vi "运维调试_五参数.vi"() -> ()   [LabVIEW 2016, in "斯坦道原位多参数.lvlib"]
uses:
  <vilib>/Utility/miscctls.llb/LVPointTypeDef.ctl
  <vilib>/Utility/config.llb/NI_LVConfig.lvlib
panel:
  in  "获取传感器参数并保存触发":bool
  in  "传感器参数自动获取":bool=TRUE
  in  "标样测试组数":dbl=1.0 caption="标样测试组数:"
  in  "水样测试组数":dbl=1.0 caption="水样测试组数:"
  in  "转刷清洗时间":dbl=30.0 caption="转刷清洗时间:"
  in  "上电初始化时间":dbl=5.0 caption="上电初始化时间:"
  in  "水样稳定时间":dbl=5.0 caption="水样稳定时间:"
  out "串口号":string
  in  "水深写入":bool
  in  "水深读取":bool
  in  "水深校准":dbl caption="水深校准:"
  out "模块版本号":string
  in  "写入":bool
  in  "读取":bool
  in  "B":dbl caption="校准值B:"
  in  "K":dbl caption="校准值K:"
  in  "标样核查":bool
  in  "串口设置":bool
  in  "质控参数设置":bool
  in  "打开串口":bool
  in  "释放串口":bool
  out "多参数横条运行状态":T1(xcontrol)
  in  "数据区":i32(listbox)
  in  "停止测量(单探)":bool
  in  "启动测量(单探)":bool
  in  "控制命令区探头选择":u16(ring)=9 items=["氨氮"=3, "水温"=9, "pH值"=10, "溶解氧"=11, "电导率"=12, "浊度"=13, "叶绿素a"=14, "藻密度"=15, "蓝绿藻"=16, "氧化还原电位"=17, "溶解氧%"=18, "盐度"=19]
  in  "同步时间":bool
  in  "初始化(清洗)":bool
  in  "停止测量(全部)":bool
  in  "启动测量(全部)":bool
  in  "关键参数区读取":bool
  in  "关键参数区":i32(listbox)
  in  "传感器参数读取":bool
  in  "传感器区":i32(listbox)
  in  "返回":bool
  in  "设置":bool
  out "运行状态":string
  in  "停止":bool
  in  "水样测试":bool
  out "集成报警信息":string
  # "min"
  # "组"
  # "组"
  # "s"
  # "s"
  # "控制命令区"
  # "探头校准"
  # "水深校准"
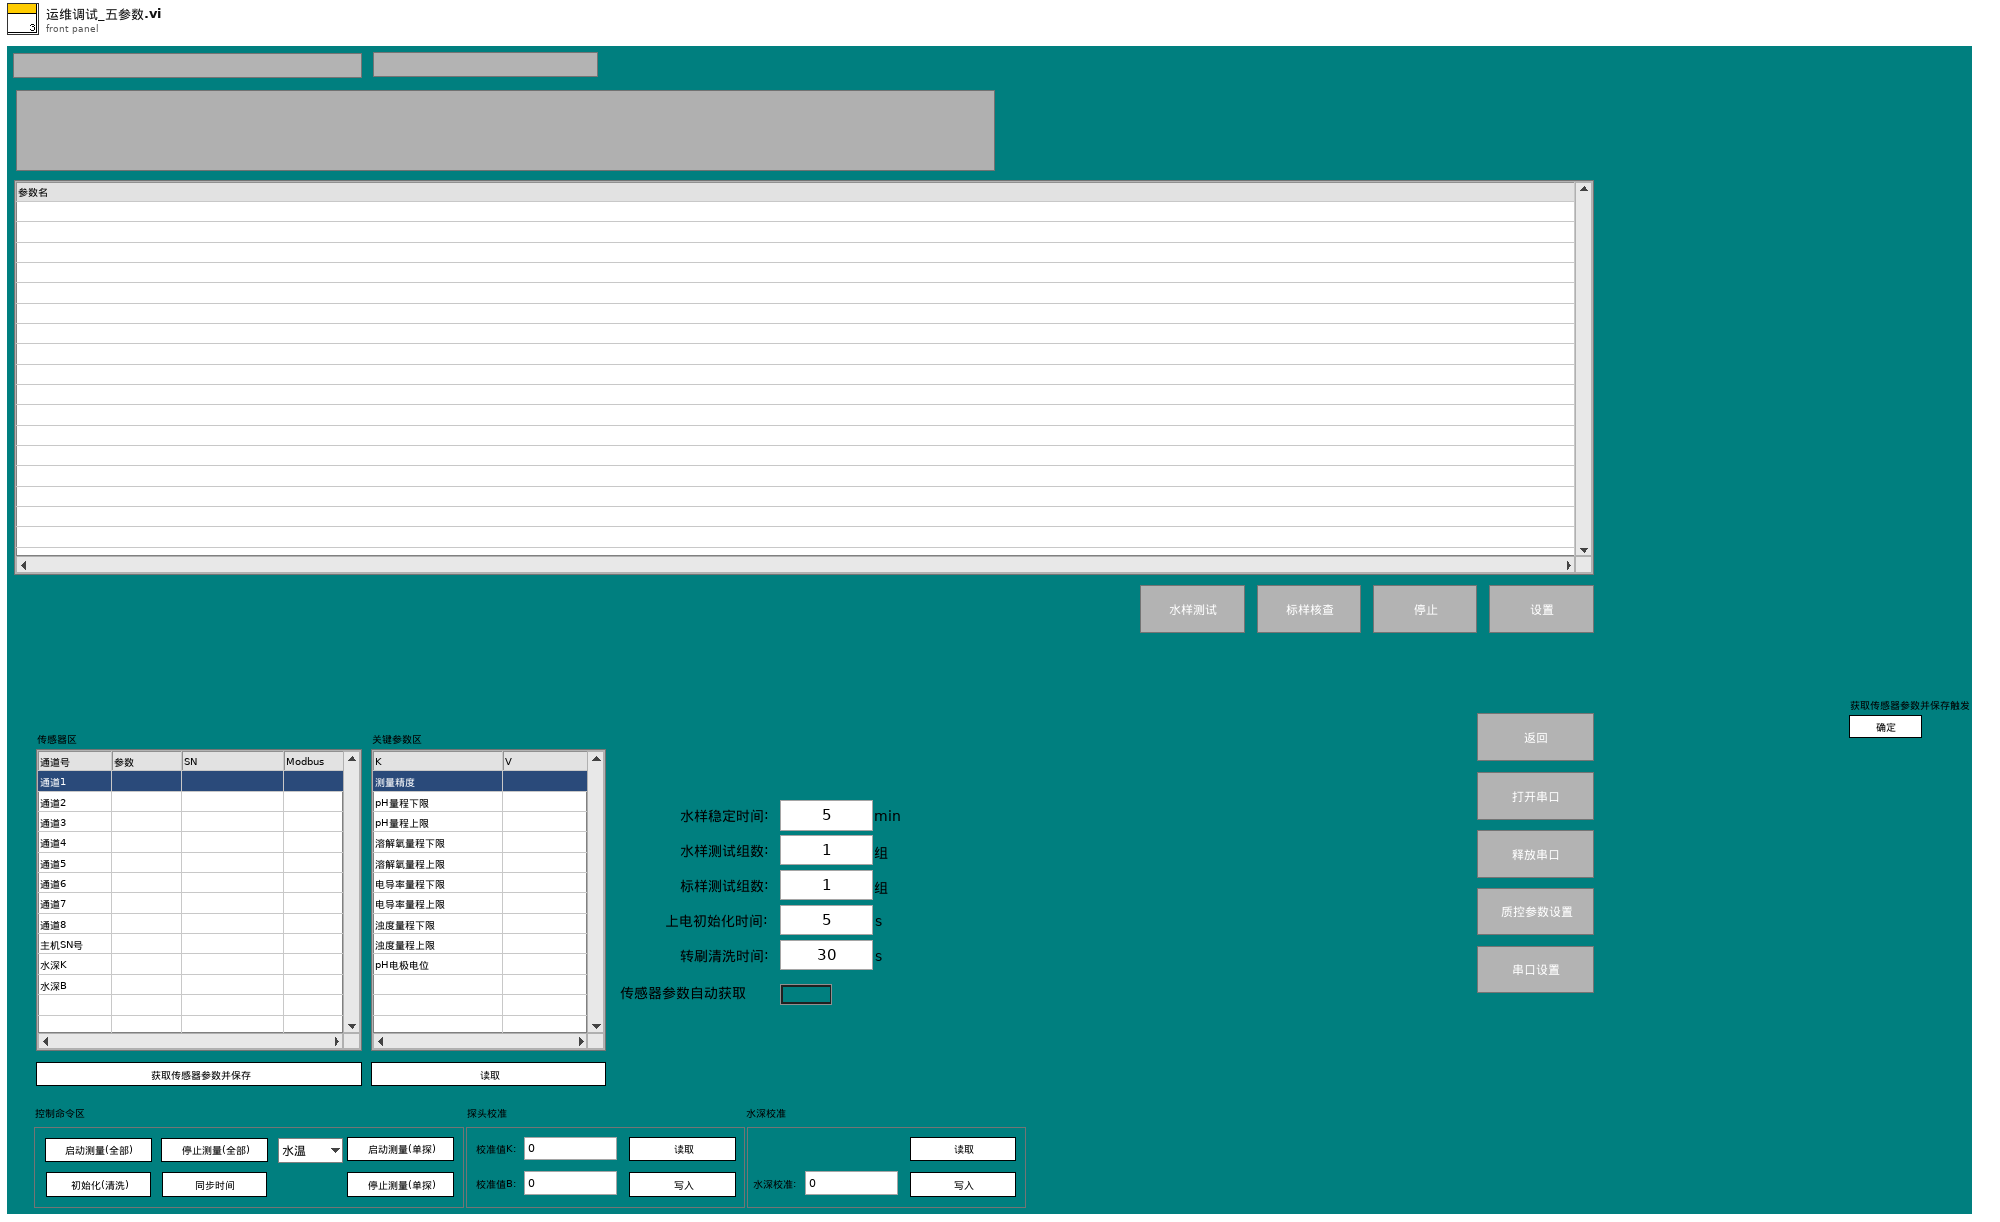
[diagram p1: front panel]
types:
  T1 = cluster{"系统时间":timestamp, "工作状态":u16, "测量模式":u16, "告警代码":enum16{"无告警", "缺试剂告警", "缺水样告警", "缺蒸馏水告警", "缺标液告警", "仪表漏液告警", "标定异常告警", "超量程告警", "加热异常", "低试剂预警", "超上限告警", "超下限告警", "仪表内部其他异常", "滴定异常告警", "电极异常告警", "量程切换告警", "参数设置告警", "PH电极电位异常", "电导率电极异常", "浊度光度异常", "溶解氧电极异常", "溶解氧光强异常", "温度异常告警", "PH异常告警", "溶解氧异常告警", "电导率异常告警", "浊度异常告警", "叶绿素异常告警", "藻密度异常告警", "蓝绿藻异常告警", "ORP异常告警", "氨氮异常告警", "清洁刷异常告警", "SD卡异常告警", "蓝牙异常告警", "Wifi异常告警", "流程异常告警"}, "故障代码":enum16{"无故障", "电机故障", "温度故障", "通讯故障", "滴定故障"}, "日志代码":u16, "软件版本":string}
  T2 = typedef "斯坦道原位多参数.lvlib/水样测试启动自定义输入参数.ctl" = cluster{"测量模式":string, "数据类型":string}
  T3 = typedef "LVPointTypeDef.ctl" = cluster{"Horizontal":i16, "Vertical":i16}
  T4 = typedef "报警信息字段定义.ctl" = cluster{"时间":timestamp, "参数":string, "报警信息":string, "备注":string}
  T5 = enum16{"无告警", "缺试剂告警", "缺水样告警", "缺蒸馏水告警", "缺标液告警", "仪表漏液告警", "标定异常告警", "超量程告警", "加热异常", "低试剂预警", "超上限告警", "超下限告警", "仪表内部其他异常", "滴定异常告警", "电极异常告警", "量程切换告警", "参数设置告警", "PH电极电位异常", "电导率电极异常", "浊度光度异常", "溶解氧电极异常", "溶解氧光强异常", "温度异常告警", "PH异常告警", "溶解氧异常告警", "电导率异常告警", "浊度异常告警", "叶绿素异常告警", "藻密度异常告警", "蓝绿藻异常告警", "ORP异常告警", "氨氮异常告警", "清洁刷异常告警", "SD卡异常告警", "蓝牙异常告警", "Wifi异常告警", "流程异常告警"}
  T6 = cluster{"水温":dbl, "pH":dbl, "DO":dbl, "Cond":dbl, "Turb":dbl, "叶绿素":dbl, "藻密度":dbl, "蓝绿藻":dbl, "ORP":dbl, "NH3N":dbl}
  T7 = cluster{"因子编码":string, "单位":string, "标样参考值":sgl, "水样数据时间":timestamp, "水样实测值":sgl, "水样数据标识":string, "K":sgl, "B":sgl, "T":sgl, "H":sgl, "水深":sgl, "探头温度":sgl}
  T8 = cluster{"Major":u16, "Minor":u16, "Fix":u16, "Build":u16}
  T9 = typedef "NI_LVConfig.lvlib/Config Data RefNum.ctl" = refnum<k1>
  T10 = enum8{"Enabled", "Disabled", "Disabled and Grayed Out"}
  T11 = typedef "斯坦道原位多参数.lvlib/标样核查启动自定义输入参数.ctl" = cluster{"测量模式":string, "数据类型":string, "输出参数":cluster{"水温":bool, "pH":bool, "DO":bool, "浊度":bool, "电导率":bool}}
  T12 = cluster{"水温标准液标准浓度":dbl, "酸碱度标准液标准浓度":dbl, "溶解氧标准液标准浓度":dbl, "电导率标准液标准浓度":dbl, "浊度标准液标准浓度":dbl}
  T13 = cluster{"确定":bool, "水温标准液标准浓度":dbl, "酸碱度标准液标准浓度":dbl, "溶解氧标准液标准浓度":dbl, "电导率标准液标准浓度":dbl, "浊度标准液标准浓度":dbl}
  T14 = cluster{"运行模式":enum16{"维护模式", "常规模式", "应急模式", "质控模式"}, "24H周期设置":bool[]}
  T15 = cluster{"水温":bool, "pH":bool, "DO":bool, "浊度":bool, "电导率":bool}
  T16 = enum32{"Bad", "Idle", "Run top level", "Running"}
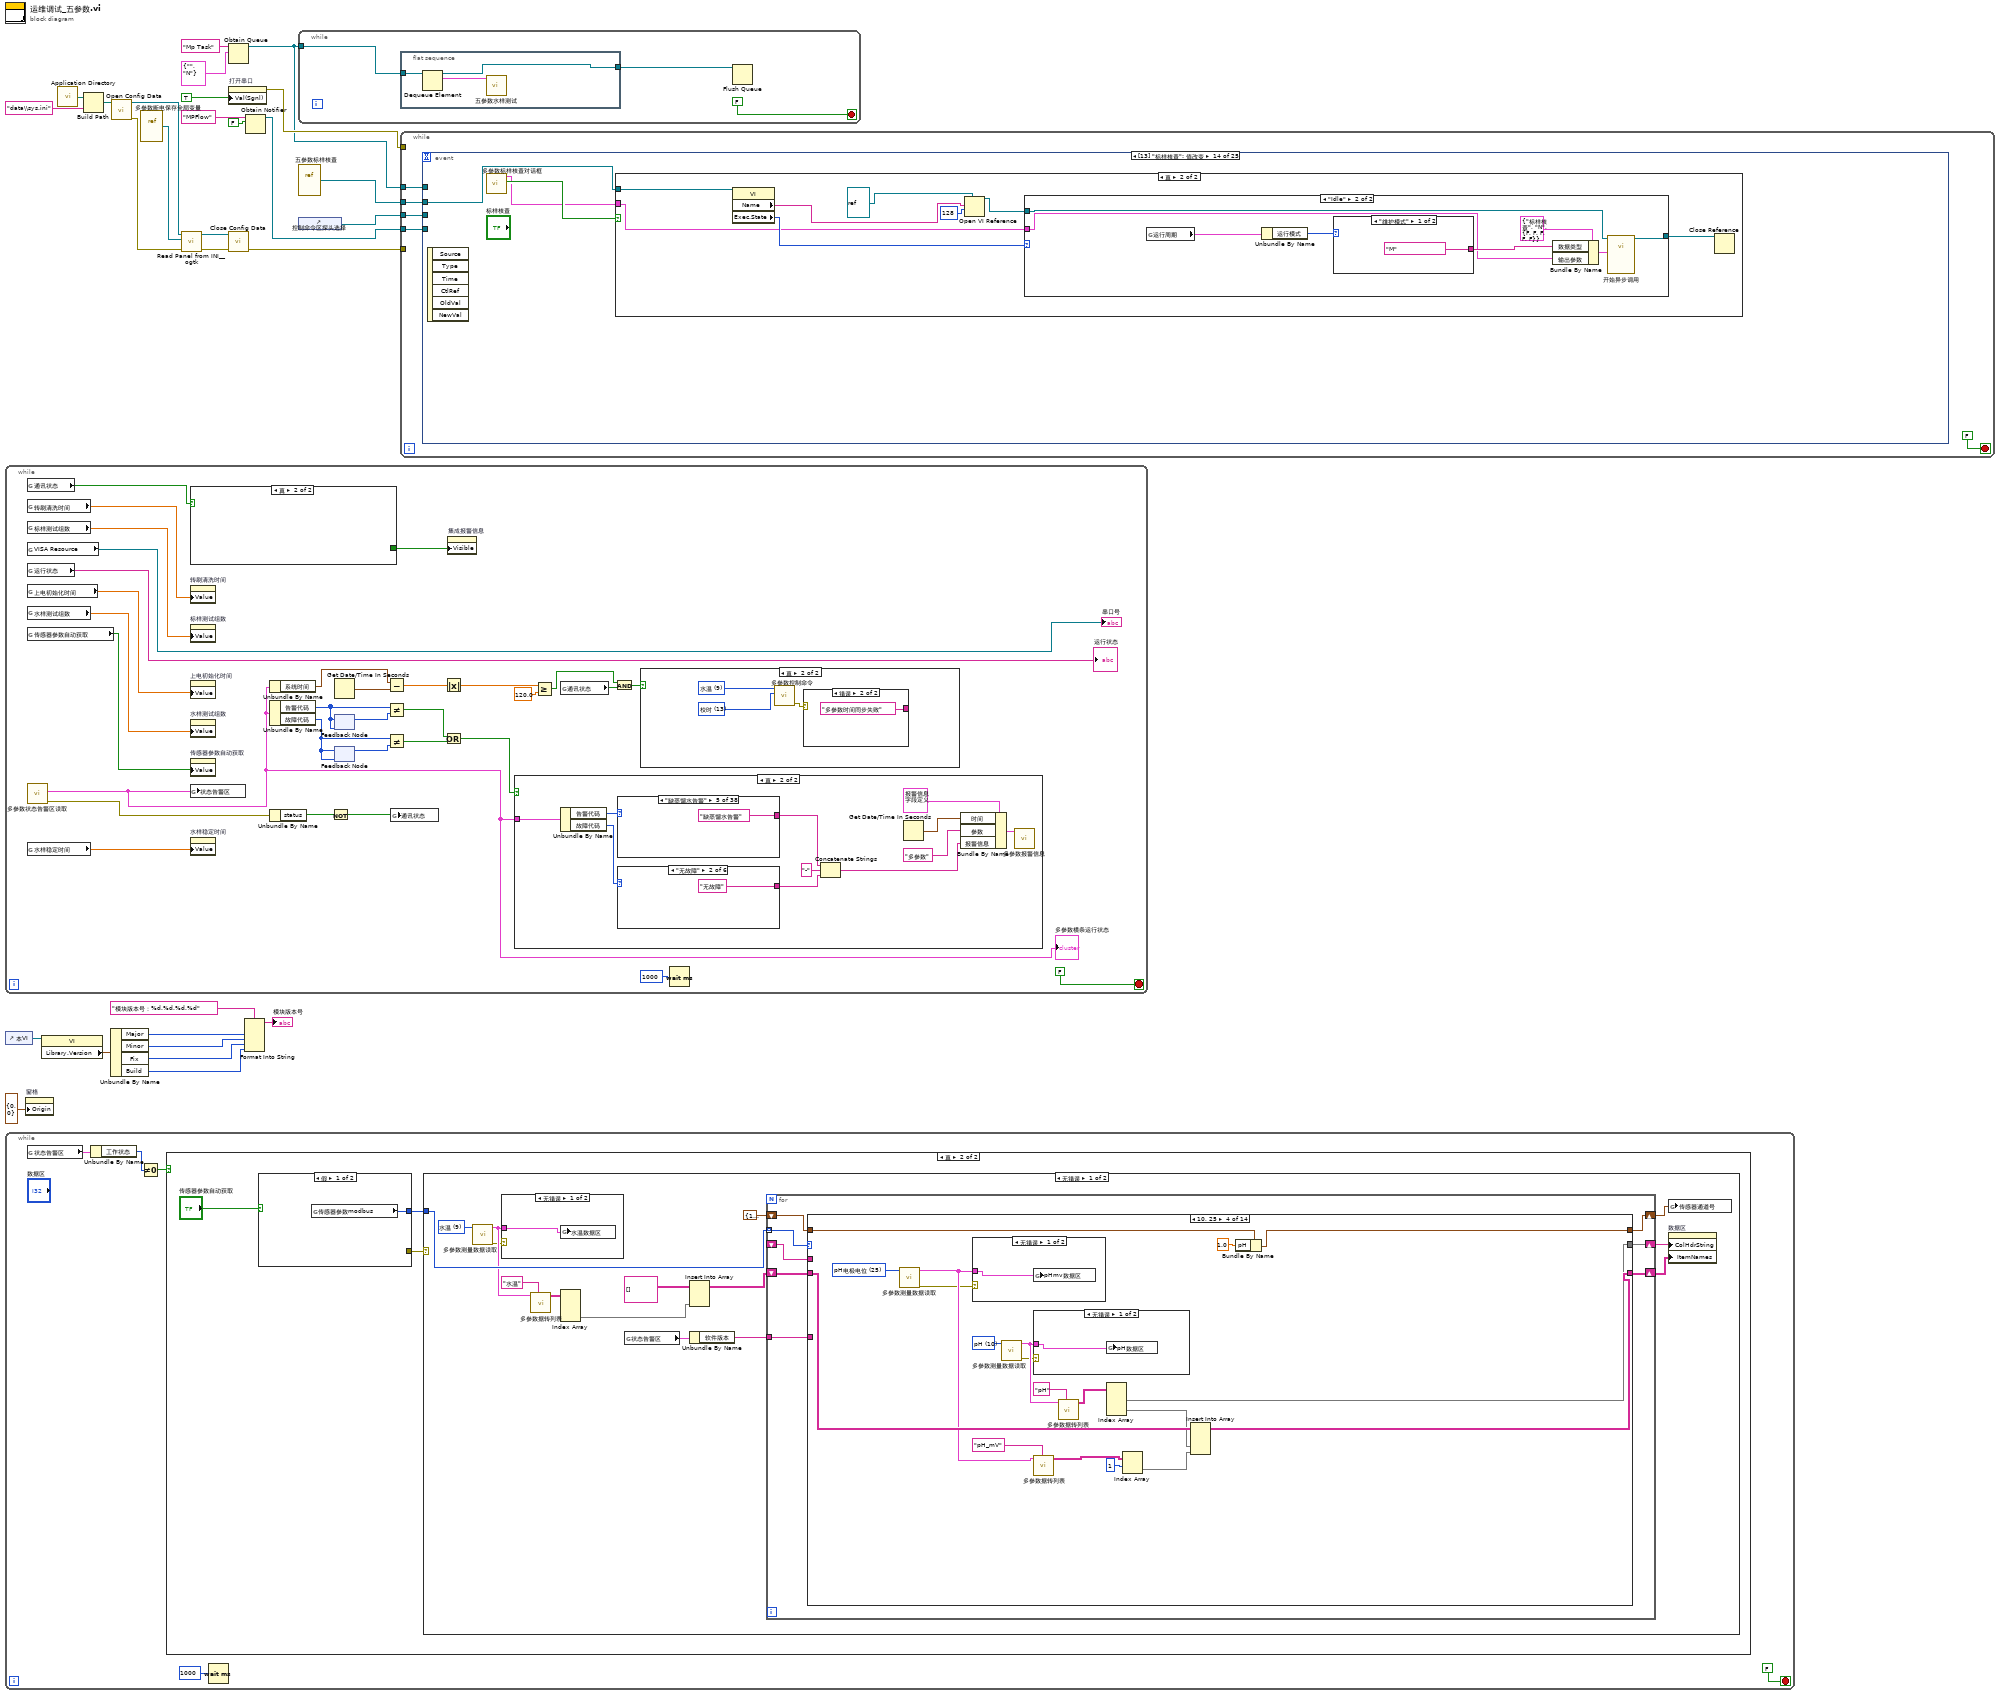
[diagram p0: block diagram]
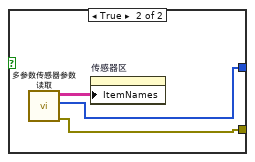
[diagram p3: hidden frame]
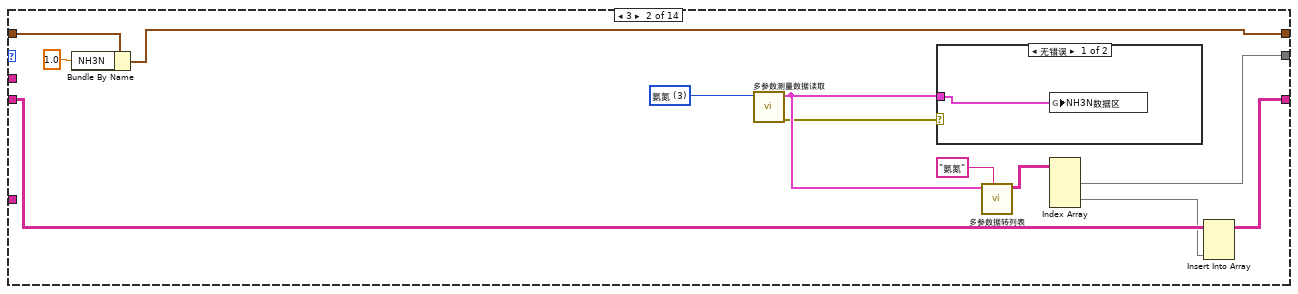
[diagram p6: hidden frame]
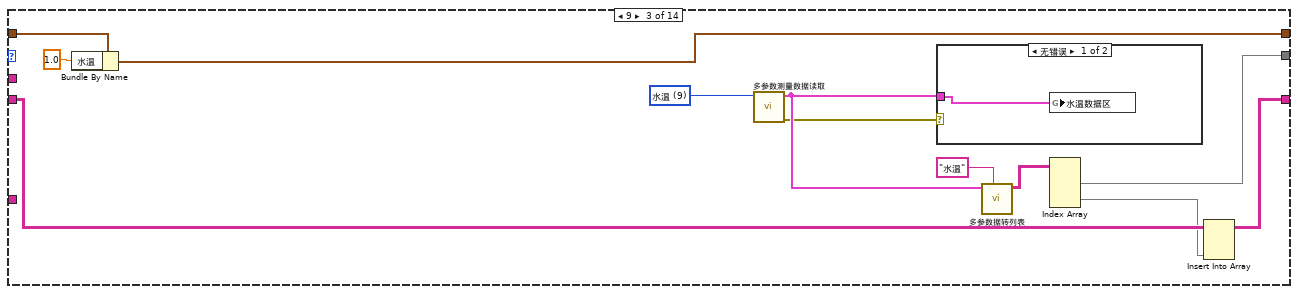
[diagram p8: hidden frame]
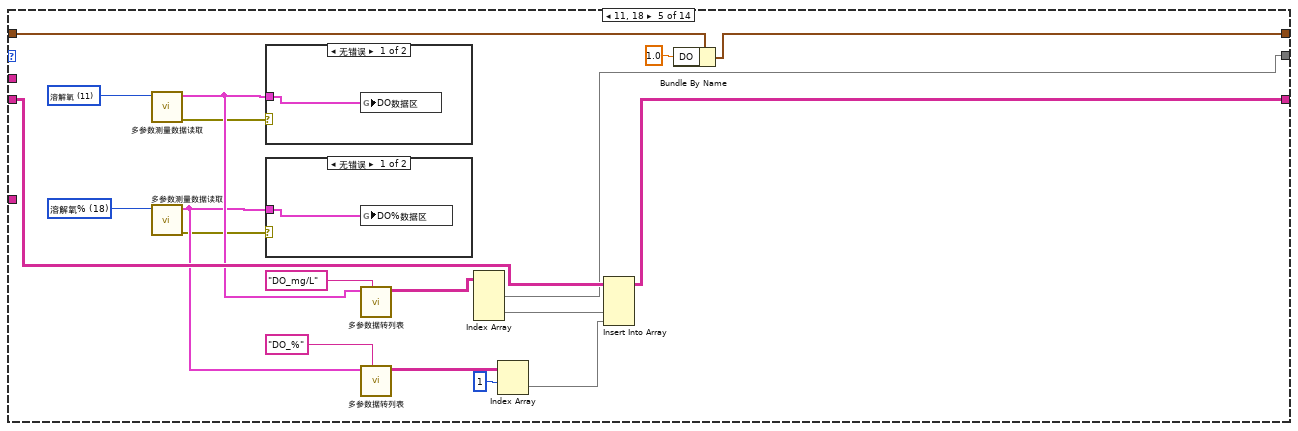
[diagram p12: hidden frame]
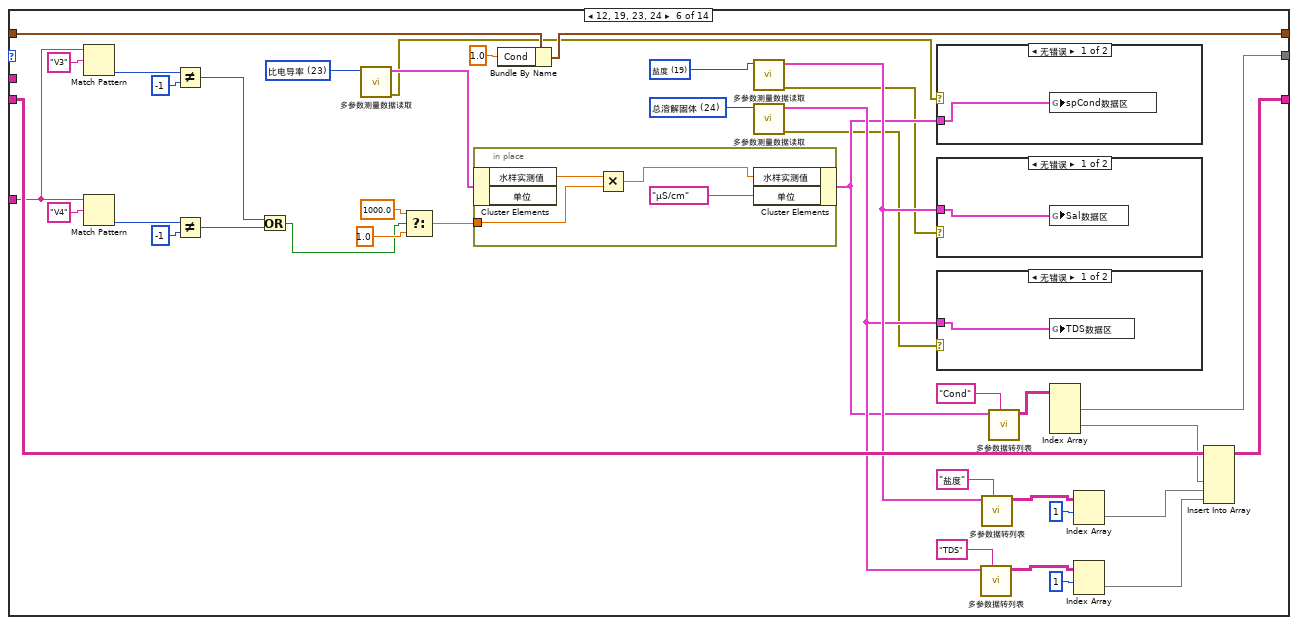
[diagram p15: hidden frame]
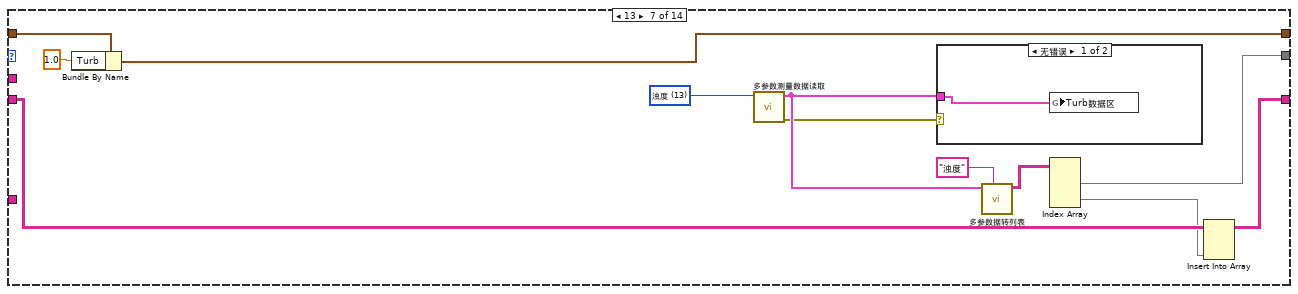
[diagram p19: hidden frame]
diagram:
  n1 = while {
    stop <- FALSE stop-if-true
    n2 = global read "多参数全局变量.vi" "通讯状态"() -> (w57:bool)
    n3 = global read "多参数断电保存全局变量.vi" "转刷清洗时间"() -> (w31:dbl)
    n4 = global read "多参数断电保存全局变量.vi" "标样测试组数"() -> (w30:dbl)
    n5 = global read "多参数断电保存全局变量.vi" "VISA Resource"() -> (→"串口号":refnum<visa-resource-name>)
    n6 = global read "多参数全局变量.vi" "运行状态"() -> (→"运行状态":string)
    n7 = global read "多参数断电保存全局变量.vi" "上电初始化时间"() -> (w32:dbl)
    n8 = global read "多参数断电保存全局变量.vi" "水样测试组数"() -> (w33:dbl)
    n9 = global read "多参数断电保存全局变量.vi" "传感器参数自动获取"() -> (w29:bool)
    n10 = call "多参数状态告警区读取.vi"() -> ("error out"=w47:errorcluster, "状态告警块"=w44:T1)  [unwired: 9 in, 1 out]
    "多参数横条运行状态" <- w44
    n11 = global read "多参数断电保存全局变量.vi" "水样稳定时间"() -> (w34:dbl)
    n12 = case shown="真" w57 {
      tunnel: [TRUE ("可见") _] -> w56
      frame False {
        "集成报警信息" <- "通讯异常" ("集成报警信息")
      }
      frame True {
      }
    }
    n13 = property on="转刷清洗时间" class="DigNum (严格)"("Value"=w31) -> ()  [unwired: 2 in, 2 out]
    n14 = property on="标样测试组数" class="DigNum (严格)"("Value"=w30) -> ()  [unwired: 2 in, 2 out]
    n15 = property on="上电初始化时间" class="DigNum (严格)"("Value"=w32) -> ()  [unwired: 2 in, 2 out]
    n16 = property on="水样测试组数" class="DigNum (严格)"("Value"=w33) -> ()  [unwired: 2 in, 2 out]
    n17 = property on="传感器参数自动获取" class="Bool (严格)"("Value"=w29) -> ()  [unwired: 2 in, 2 out]
    n18 = global write "多参数全局变量.vi" "状态告警区"(w44) -> ()
    n19 = property on="水样稳定时间" class="DigNum (严格)"("Value"=w34) -> ()  [unwired: 2 in, 2 out]
    n20 = Unbundle By Name(w44) -> ("系统时间"=w43:timestamp)
    n21 = Unbundle By Name(w44) -> ("告警代码"=w53:T5, "故障代码"=w51:enum16{"无故障", "电机故障", "温度故障", "通讯故障", "滴定故障"})
    n22 = Unbundle By Name(w47) -> ("status"=w46:bool)
    n23 = Not(x=w46) -> (.not. x?=w45:bool)
    n24 = Get Date/Time In Seconds() -> (seconds since 1Jan1904=w42:timestamp)
    n25 = feedback #1(w53) -> (w54:T5)
    n26 = feedback-in #1(w53) -> ()
    n27 = feedback #2(w51) -> (w52:enum16{"无故障", "电机故障", "温度故障", "通讯故障", "滴定故障"})
    n28 = feedback-in #2(w51) -> ()
    n29 = Subtract(x=w43, y=w42) -> (x-y=w41:dbl)
    n30 = Not Equal?(x=w53, y=w54) -> (x != y?=w49:bool)
    n31 = Not Equal?(x=w51, y=w52) -> (x != y?=w50:bool)
    n32 = global write "多参数全局变量.vi" "通讯状态"(w45) -> ()
    n33 = Absolute Value(x=w41) -> (abs(x)=w40:dbl)
    n34 = Or(x=w49, y=w50) -> (x .or. y?=w48:bool)
    n35 = property on="集成报警信息" class="Str"("Visible"=w56) -> ()  [unwired: 2 in, 2 out]
    n36 = case shown="真" w48 {
      tunnel: w44 -> [_ w75]
      frame False {
      }
      frame True {
        n37 = Unbundle By Name(w75) -> ("告警代码"=w74:T5, "故障代码"=w73:enum16{"无故障", "电机故障", "温度故障", "通讯故障", "滴定故障"})
        n38 = case shown="\"缺蒸馏水告警\"" w74 {
          selector: w74 -> [w86 _ _ _ _ _ _ _ _ _ _ _ _ _ _ _ _ _ _ _ _ _ _ _ _ _ _ _ _ _ _ _ _ _ _ _ _ _]
          tunnel: [w85 "无告警" "缺试剂告警" "缺水样告警" "缺蒸馏水告警" "缺标液告警" "仪表漏液告警" "标定异常告警" "超量程告警" "加热异常" "低试剂预警" "超上限告警" "超下限告警" "仪表内部其他异常" "滴定异常告警" "电极异常告警" "量程切换告警" "参数设置告警" "PH电极电位异常" "电导率电极异常" "浊度光度异常" "溶解氧电极异常" "溶解氧光强异常" "温度异常告警" "PH异常告警" "溶解氧异常告警" "电导率异常告警" "浊度异常告警" "叶绿素异常告警" "藻密度异常告警" "蓝绿藻异常告警" "ORP异常告警" "氨氮异常告警" "清洁刷异常告警" "SD卡异常告警" "蓝牙异常告警" "WiFi异常告警" "流程异常告警"] -> w72
          frame Default {
            n39 = Format Into String(format string="%d" ("格式字符串"), initial string="未知" ("工作状态"), w86) -> (resulting string=w85:string)  [unwired: 1 in, 1 out]
          }
          frame "无告警" {
          }
          frame "缺试剂告警" {
          }
          frame "缺水样告警" {
          }
          frame "缺蒸馏水告警" {
          }
          frame "缺标液告警" {
          }
          frame "仪表漏液告警" {
          }
          frame "标定异常告警" {
          }
          frame "超量程告警" {
          }
          frame "加热异常" {
          }
          frame "低试剂预警" {
          }
          frame "超上限告警" {
          }
          frame "超下限告警" {
          }
          frame "仪表内部其他异常" {
          }
          frame "滴定异常告警" {
          }
          frame "电极异常告警" {
          }
          frame "量程切换告警" {
          }
          frame "参数设置告警" {
          }
          frame "PH电极电位异常" {
          }
          frame "电导率电极异常" {
          }
          frame "浊度光度异常" {
          }
          frame "溶解氧电极异常" {
          }
          frame "溶解氧光强异常" {
          }
          frame "温度异常告警" {
          }
          frame "PH异常告警" {
          }
          frame "溶解氧异常告警" {
          }
          frame "电导率异常告警" {
          }
          frame "浊度异常告警" {
          }
          frame "叶绿素异常告警" {
          }
          frame "藻密度异常告警" {
          }
          frame "蓝绿藻异常告警" {
          }
          frame "ORP异常告警" {
          }
          frame "氨氮异常告警" {
          }
          frame "清洁刷异常告警" {
          }
          frame "SD卡异常告警" {
          }
          frame "蓝牙异常告警" {
          }
          frame "Wifi异常告警" {
          }
          frame "流程异常告警" {
          }
        }
        n40 = case shown="\"无故障\"" w73 {
          selector: w73 -> [w77 _ _ _ _ _]
          tunnel: [w76 "无故障" "电机故障" "温度故障" "通讯故障" "滴定故障"] -> w71
          frame Default {
            n41 = Format Into String(format string="%d" ("格式字符串"), initial string="未知" ("工作状态"), w77) -> (resulting string=w76:string)  [unwired: 1 in, 1 out]
          }
          frame "无故障" {
          }
          frame "电机故障" {
          }
          frame "温度故障" {
          }
          frame "通讯故障" {
          }
          frame "滴定故障" {
          }
        }
        n42 = Concatenate Strings(w72, "-" ("字符串"), w71) -> (w69:string)
        n43 = Get Date/Time In Seconds() -> (seconds since 1Jan1904=w68:timestamp)
        n44 = Bundle By Name(cluster=T4 {"时间"=timestamp(0 s since 1904-01-01), "参数"="", "报警信息"="", "备注"=""} ("data"), "时间"=w68, "参数"="多参数" ("设备"), "报警信息"=w69) -> (w65:T4)
        n45 = call "多参数报警信息.vi"("data"=w65) -> ()  [unwired: 10 in, 1 out]
      }
    }
    n46 = Greater Or Equal?(x=w40, y=120.0) -> (x >= y?=w39:bool)
    n47 = global read "多参数全局变量.vi" "通讯状态"() -> (w36:bool)
    n48 = And(x=w39, y=w36) -> (x .and. y?=w37:bool)
    n49 = case shown="真" w37 {
      frame False {
      }
      frame True {
        w60 = u16 13 items=["启动测量（全部）"=1, "初始化（清洗）"=10, "停止测量（全部）"=11, "校时"=13, "启动测量（单个传感器）"=19, "停止测量（单个传感器）"=20] ("控制命令")
        w61 = u16 9 items=["氨氮"=3, "水温"=9, "pH值"=10, "溶解氧"=11, "电导率"=12, "浊度"=13, "叶绿素a"=14, "藻密度"=15, "蓝绿藻"=16, "氧化还原电位"=17, "溶解氧%"=18, "盐度"=19] ("站号")
        n50 = call "多参数控制命令.vi"("控制命令"=w60, "站号"=w61) -> ("error out"=w62:errorcluster)  [unwired: 9 in]
        n51 = case shown="错误" w62 {
          tunnel: ["多参数时间同步成功" ("消息") "多参数时间同步失败" ("消息")] -> _
          frame No Error {
          }
          frame Error {
          }
        }
      }
    }
    n52 = Wait (ms)(milliseconds to wait=u32 1000 ("等待时间（毫秒）")) -> ()  [unwired: 1 out]
  }
  n53 = control-ref of="本VI"() -> (w8:refnum<vi>)
  n54 = while {
    stop <- FALSE stop-if-true
    n55 = global read "多参数全局变量.vi" "状态告警区"() -> (w130:T1)
    n56 = Unbundle By Name(w130) -> ("工作状态"=w129:u16)
    n57 = Not Equal To 0?(x=w129) -> (x != 0?=w128:bool)
    n58 = case shown="真" w128 {
      frame False {
      }
      frame True {
        n59 = case shown="假" "传感器参数自动获取" {
          tunnel: [_ w139] -> w135
          tunnel: [w136 w138] -> w134
          frame False {
            n60 = global read "多参数断电保存全局变量.vi" "传感器参数modbus"() -> (w136:u16[])
          }
          frame True {
            n61 = call "多参数传感器参数读取.vi"() -> ("error out"=w139:errorcluster, "modbus"=w138:u16[], "添加的数组"=w137:string[][])  [unwired: 9 in]
            n62 = property on="传感器区" class="MCListbox (严格)"("ItemNames"=w137) -> ()  [unwired: 2 in, 2 out]
          }
        }
        n63 = case shown="无错误" w135 {
          tunnel: w134 -> [w154 _]
          frame No Error {
            w151 = u16 9 items=["氨氮"=3, "水温"=9, "pH"=10, "溶解氧"=11, "电导率"=12, "浊度"=13, "叶绿素a"=14, "藻密度"=15, "蓝绿藻"=16, "氧化还原电位"=17, "溶解氧%"=18, "盐度"=19, "水中油"=20, "高锰酸盐指数"=21, "化学需氧量"=22, "比电导率"=23, "总溶解固体"=24, "pH电极电位"=25] ("下拉列表")
            n64 = call "多参数测量数据读取.vi"("探头选择"=w151) -> ("error out"=w140:errorcluster, "测量数据块"=w146:T7)  [unwired: 8 in, 1 out]
            n65 = case shown="无错误" w140 {
              tunnel: w146 -> [w155 _]
              frame No Error {
                n66 = global write "多参数全局变量.vi" "水温数据区"(w155) -> ()
              }
              frame Error {
              }
            }
            n67 = call "多参数据转列表.vi"("参数名"="水温", "测量数据块"=w146) -> ("添加的数组"=w144:string[][])  [unwired: 9 in]
            n68 = Index Array(array=w144) -> (element #2=w143:string[])  [unwired: 4 in, 1 out]
            n69 = global read "多参数全局变量.vi" "状态告警区"() -> (w142:T1)
            n70 = Insert Into Array(array=string[][] [] ("子数组"), new element=w143) -> (w149:string[][])  [unwired: 2 in]
            n71 = Unbundle By Name(w142) -> ("软件版本"=w141:string)
            n72 = for {
              tunnel: w154 -> [w163] mode=indexing
              shift-right: [w161] -> w152
              shift-left: w149 -> [w162]
              shift-right: [w160] -> w153
              shift-left: _ -> [w159]
              shift-right: [w158] -> w147
              shift-left: T6 {"水温"=1.0, "pH"=0.0, "DO"=0.0, "Cond"=0.0, "Turb"=0.0, "叶绿素"=0.0, "藻密度"=0.0, "蓝绿藻"=0.0, "ORP"=0.0, "NH3N"=0.0} ("传感器通道号") -> [w157]
              tunnel: w141 -> [w156]
              n73 = case shown="10, 25" w163 {
                tunnel: w162 -> [w166 w177 w190 w210 w231 w273 w292 w305 w318 w331 w344 w354 w363 w372]
                tunnel: [w166 w176 w189 w209 w230 w272 w291 w304 w317 w330 w343 w353 w362 w371] -> w161
                tunnel: [w165 w169 w182 w202 w223 w264 w285 w297 w312 w324 w337 w348 w357 w366] -> w160
                tunnel: w159 -> [w165 _ _ _ _ _ _ _ _ _ _ _ _ _]
                tunnel: [w164 w173 w186 w205 w227 w267 w288 w301 w314 w327 w340 w352 w361 w370] -> w158
                tunnel: w157 -> [w164 w175 w188 w207 w229 w268 w289 w302 w315 w328 w341 w352 w361 w370]
                tunnel: w156 -> [_ _ _ _ _ w243 _ _ _ _ _ _ _ _]
                frame 0, Default {
                }
                frame 3 {
                  w178 = u16 3 items=["氨氮"=3, "水温"=9, "pH"=10, "溶解氧"=11, "电导率"=12, "浊度"=13, "叶绿素a"=14, "藻密度"=15, "蓝绿藻"=16, "氧化还原电位"=17, "溶解氧%"=18, "盐度"=19, "水中油"=20, "高锰酸盐指数"=21, "化学需氧量"=22, "比电导率"=23, "总溶解固体"=24, "pH电极电位"=25] ("下拉列表")
                  n74 = Bundle By Name(cluster=w175, "NH3N"=1.0) -> (w173:T6)
                  n75 = call "多参数测量数据读取.vi"("探头选择"=w178) -> ("error out"=w167:errorcluster, "测量数据块"=w172:T7)  [unwired: 8 in, 1 out]
                  n76 = case shown="无错误" w167 {
                    tunnel: w172 -> [w179 _]
                    frame No Error {
                      n77 = global write "多参数全局变量.vi" "NH3N数据区"(w179) -> ()
                    }
                    frame Error {
                    }
                  }
                  n78 = call "多参数据转列表.vi"("参数名"="氨氮", "测量数据块"=w172) -> ("添加的数组"=w171:string[][])  [unwired: 9 in]
                  n79 = Index Array(array=w171) -> (element #1=w169:string[], element #2=w168:string[])  [unwired: 4 in]
                  n80 = Insert Into Array(array=w177, new element=w168) -> (w176:string[][])  [unwired: 2 in]
                }
                frame 9 {
                  w191 = u16 9 items=["氨氮"=3, "水温"=9, "pH"=10, "溶解氧"=11, "电导率"=12, "浊度"=13, "叶绿素a"=14, "藻密度"=15, "蓝绿藻"=16, "氧化还原电位"=17, "溶解氧%"=18, "盐度"=19, "水中油"=20, "高锰酸盐指数"=21, "化学需氧量"=22, "比电导率"=23, "总溶解固体"=24, "pH电极电位"=25] ("下拉列表")
                  n81 = Bundle By Name(cluster=w188, "水温"=1.0) -> (w186:T6)
                  n82 = call "多参数测量数据读取.vi"("探头选择"=w191) -> ("error out"=w180:errorcluster, "测量数据块"=w185:T7)  [unwired: 8 in, 1 out]
                  n83 = case shown="无错误" w180 {
                    tunnel: w185 -> [w192 _]
                    frame No Error {
                      n84 = global write "多参数全局变量.vi" "水温数据区"(w192) -> ()
                    }
                    frame Error {
                    }
                  }
                  n85 = call "多参数据转列表.vi"("参数名"="水温", "测量数据块"=w185) -> ("添加的数组"=w184:string[][])  [unwired: 9 in]
                  n86 = Index Array(array=w184) -> (element #1=w182:string[], element #2=w181:string[])  [unwired: 4 in]
                  n87 = Insert Into Array(array=w190, new element=w181) -> (w189:string[][])  [unwired: 2 in]
                }
                frame 10, 25 {
                  w208 = u16 25 items=["氨氮"=3, "水温"=9, "pH"=10, "溶解氧"=11, "电导率"=12, "浊度"=13, "叶绿素a"=14, "藻密度"=15, "蓝绿藻"=16, "氧化还原电位"=17, "溶解氧%"=18, "盐度"=19, "水中油"=20, "高锰酸盐指数"=21, "化学需氧量"=22, "比电导率"=23, "总溶解固体"=24, "pH电极电位"=25] ("下拉列表")
                  w211 = u16 10 items=["氨氮"=3, "水温"=9, "pH"=10, "溶解氧"=11, "电导率"=12, "浊度"=13, "叶绿素a"=14, "藻密度"=15, "蓝绿藻"=16, "氧化还原电位"=17, "溶解氧%"=18, "盐度"=19, "水中油"=20, "高锰酸盐指数"=21, "化学需氧量"=22, "比电导率"=23, "总溶解固体"=24, "pH电极电位"=25] ("下拉列表")
                  n88 = call "多参数测量数据读取.vi"("探头选择"=w208) -> ("error out"=w193:errorcluster, "测量数据块"=w198:T7)  [unwired: 8 in, 1 out]
                  n89 = case shown="无错误" w193 {
                    tunnel: w198 -> [w212 _]
                    frame No Error {
                      n90 = global write "多参数全局变量.vi" "pHmv数据区"(w212) -> ()
                    }
                    frame Error {
                    }
                  }
                  n91 = call "多参数测量数据读取.vi"("探头选择"=w211) -> ("error out"=w194:errorcluster, "测量数据块"=w204:T7)  [unwired: 8 in, 1 out]
                  n92 = case shown="无错误" w194 {
                    tunnel: w204 -> [w213 _]
                    frame No Error {
                      n93 = global write "多参数全局变量.vi" "pH数据区"(w213) -> ()
                    }
                    frame Error {
                    }
                  }
                  n94 = call "多参数据转列表.vi"("参数名"="pH_mV", "测量数据块"=w198) -> ("添加的数组"=w197:string[][])  [unwired: 9 in]
                  n95 = call "多参数据转列表.vi"("参数名"="pH", "测量数据块"=w204) -> ("添加的数组"=w203:string[][])  [unwired: 9 in]
                  n96 = Index Array(array=w203) -> (element #1=w202:string[], element #2=w201:string[])  [unwired: 4 in]
                  n97 = Index Array(array=w197, index (row)=1 ("禁用的索引 (列)")) -> (element=w200:string[])  [unwired: 1 in]
                  n98 = Insert Into Array(array=w210, new element #1=w201, new element #2=w200) -> (w209:string[][])  [unwired: 2 in]
                  n99 = Bundle By Name(cluster=w207, "pH"=1.0) -> (w205:T6)
                }
                frame 11, 18 {
                  w221 = u16 18 items=["氨氮"=3, "水温"=9, "pH"=10, "溶解氧"=11, "电导率"=12, "浊度"=13, "叶绿素a"=14, "藻密度"=15, "蓝绿藻"=16, "氧化还原电位"=17, "溶解氧%"=18, "盐度"=19, "水中油"=20, "高锰酸盐指数"=21, "化学需氧量"=22, "比电导率"=23, "总溶解固体"=24, "pH电极电位"=25] ("下拉列表")
                  w232 = u16 11 items=["氨氮"=3, "水温"=9, "pH"=10, "溶解氧"=11, "电导率"=12, "浊度"=13, "叶绿素a"=14, "藻密度"=15, "蓝绿藻"=16, "氧化还原电位"=17, "溶解氧%"=18, "盐度"=19, "水中油"=20, "高锰酸盐指数"=21, "化学需氧量"=22, "比电导率"=23, "总溶解固体"=24, "pH电极电位"=25] ("下拉列表")
                  n100 = call "多参数测量数据读取.vi"("探头选择"=w232) -> ("error out"=w215:errorcluster, "测量数据块"=w226:T7)  [unwired: 8 in, 1 out]
                  n101 = call "多参数测量数据读取.vi"("探头选择"=w221) -> ("error out"=w214:errorcluster, "测量数据块"=w220:T7)  [unwired: 8 in, 1 out]
                  n102 = case shown="无错误" w215 {
                    tunnel: w226 -> [w234 _]
                    frame No Error {
                      n103 = global write "多参数全局变量.vi" "DO数据区"(w234) -> ()
                    }
                    frame Error {
                    }
                  }
                  n104 = case shown="无错误" w214 {
                    tunnel: w220 -> [w233 _]
                    frame No Error {
                      n105 = global write "多参数全局变量.vi" "DO%数据区"(w233) -> ()
                    }
                    frame Error {
                    }
                  }
                  n106 = call "多参数据转列表.vi"("参数名"="DO_mg/L", "测量数据块"=w226) -> ("添加的数组"=w224:string[][])  [unwired: 9 in]
                  n107 = call "多参数据转列表.vi"("参数名"="DO_%", "测量数据块"=w220) -> ("添加的数组"=w218:string[][])  [unwired: 9 in]
                  n108 = Index Array(array=w224) -> (element #1=w223:string[], element #2=w222:string[])  [unwired: 4 in]
                  n109 = Index Array(array=w218, index (row)=1 ("禁用的索引 (列)")) -> (element=w217:string[])  [unwired: 1 in]
                  n110 = Insert Into Array(array=w231, new element #1=w222, new element #2=w217) -> (w230:string[][])  [unwired: 2 in]
                  n111 = Bundle By Name(cluster=w229, "DO"=1.0) -> (w227:T6)
                }
                frame 12, 19, 23, 24 {
                  w270 = u16 24 items=["氨氮"=3, "水温"=9, "pH"=10, "溶解氧"=11, "电导率"=12, "浊度"=13, "叶绿素a"=14, "藻密度"=15, "蓝绿藻"=16, "氧化还原电位"=17, "溶解氧%"=18, "盐度"=19, "水中油"=20, "高锰酸盐指数"=21, "化学需氧量"=22, "比电导率"=23, "总溶解固体"=24, "pH电极电位"=25] ("下拉列表")
                  w271 = u16 19 items=["氨氮"=3, "水温"=9, "pH"=10, "溶解氧"=11, "电导率"=12, "浊度"=13, "叶绿素a"=14, "藻密度"=15, "蓝绿藻"=16, "氧化还原电位"=17, "溶解氧%"=18, "盐度"=19, "水中油"=20, "高锰酸盐指数"=21, "化学需氧量"=22, "比电导率"=23, "总溶解固体"=24, "pH电极电位"=25] ("下拉列表")
                  w274 = u16 23 items=["氨氮"=3, "水温"=9, "pH"=10, "溶解氧"=11, "电导率"=12, "浊度"=13, "叶绿素a"=14, "藻密度"=15, "蓝绿藻"=16, "氧化还原电位"=17, "溶解氧%"=18, "盐度"=19, "水中油"=20, "高锰酸盐指数"=21, "化学需氧量"=22, "比电导率"=23, "总溶解固体"=24, "pH电极电位"=25] ("下拉列表")
                  n112 = Match Pattern(string=w243, regular expression="V3" ("正则表达式")) -> (offset past match=w251:i32)  [unwired: 1 in, 3 out]
                  n113 = Match Pattern(string=w243, regular expression="V4" ("正则表达式")) -> (offset past match=w245:i32)  [unwired: 1 in, 3 out]
                  n114 = Not Equal?(x=w251, y=-1) -> (x != y?=w241:bool)
                  n115 = Not Equal?(x=w245, y=-1) -> (x != y?=w242:bool)
                  n116 = Or(x=w241, y=w242) -> (x .or. y?=w240:bool)
                  n117 = call "多参数测量数据读取.vi"("探头选择"=w274) -> ("error out"=w237:errorcluster, "测量数据块"=w256:T7)  [unwired: 8 in, 1 out]
                  n118 = Select(t=1000.0, s=w240, f=1.0) -> (s? t:f=w247:dbl)
                  n119 = in-place {
                    in-place-border: w247 -> [w278]
                    n120 = in-place-cluster #3(w256) -> ("水样实测值"=w280:sgl)  [unwired: 1 out]
                    n121 = Multiply(x=w280, y=w278) -> (x*y=w279:dbl)
                    n122 = in-place-cluster #3("水样实测值"=w279, "单位"="μS/cm") -> (w255:T7)
                  }
                  n123 = Bundle By Name(cluster=w268, "Cond"=1.0 ("DO")) -> (w267:T6)
                  n124 = call "多参数测量数据读取.vi"("探头选择"=w271) -> ("error out"=w236:errorcluster, "测量数据块"=w261:T7)  [unwired: 8 in, 1 out]
                  n125 = call "多参数测量数据读取.vi"("探头选择"=w270) -> ("error out"=w235:errorcluster, "测量数据块"=w258:T7)  [unwired: 8 in, 1 out]
                  n126 = case shown="无错误" w237 {
                    tunnel: w255 -> [w277 _]
                    frame No Error {
                      n127 = global write "多参数全局变量.vi" "spCond数据区"(w277) -> ()
                    }
                    frame Error {
                    }
                  }
                  n128 = case shown="无错误" w236 {
                    tunnel: w261 -> [w276 _]
                    frame No Error {
                      n129 = global write "多参数全局变量.vi" "Sal数据区"(w276) -> ()
                    }
                    frame Error {
                    }
                  }
                  n130 = case shown="无错误" w235 {
                    tunnel: w258 -> [w275 _]
                    frame No Error {
                      n131 = global write "多参数全局变量.vi" "TDS数据区"(w275) -> ()
                    }
                    frame Error {
                    }
                  }
                  n132 = call "多参数据转列表.vi"("参数名"="TDS", "测量数据块"=w258) -> ("添加的数组"=w257:string[][])  [unwired: 9 in]
                  n133 = call "多参数据转列表.vi"("参数名"="盐度", "测量数据块"=w261) -> ("添加的数组"=w260:string[][])  [unwired: 9 in]
                  n134 = call "多参数据转列表.vi"("参数名"="Cond", "测量数据块"=w255) -> ("添加的数组"=w265:string[][])  [unwired: 9 in]
                  n135 = Index Array(array=w265) -> (element #1=w264:string[], element #2=w263:string[])  [unwired: 4 in]
                  n136 = Index Array(array=w260, index (row)=1 ("禁用的索引 (列)")) -> (element=w239:string[])  [unwired: 1 in]
                  n137 = Index Array(array=w257, index (row)=1 ("禁用的索引 (列)")) -> (element=w238:string[])  [unwired: 1 in]
                  n138 = Insert Into Array(array=w273, new element #1=w263, new element #2=w239, new element #3=w238) -> (w272:string[][])  [unwired: 2 in]
                }
                frame 13 {
                  w293 = u16 13 items=["氨氮"=3, "水温"=9, "pH"=10, "溶解氧"=11, "电导率"=12, "浊度"=13, "叶绿素a"=14, "藻密度"=15, "蓝绿藻"=16, "氧化还原电位"=17, "溶解氧%"=18, "盐度"=19, "水中油"=20, "高锰酸盐指数"=21, "化学需氧量"=22, "比电导率"=23, "总溶解固体"=24, "pH电极电位"=25] ("下拉列表")
                  n139 = Bundle By Name(cluster=w289, "Turb"=1.0 ("DO")) -> (w288:T6)
                  n140 = call "多参数测量数据读取.vi"("探头选择"=w293) -> ("error out"=w282:errorcluster, "测量数据块"=w283:T7)  [unwired: 8 in, 1 out]
                  n141 = case shown="无错误" w282 {
                    tunnel: w283 -> [w294 _]
                    frame No Error {
                      n142 = global write "多参数全局变量.vi" "Turb数据区"(w294) -> ()
                    }
                    frame Error {
                    }
                  }
                  n143 = call "多参数据转列表.vi"("参数名"="浊度", "测量数据块"=w283) -> ("添加的数组"=w286:string[][])  [unwired: 9 in]
                  n144 = Index Array(array=w286) -> (element #1=w285:string[], element #2=w284:string[])  [unwired: 4 in]
                  n145 = Insert Into Array(array=w292, new element=w284) -> (w291:string[][])  [unwired: 2 in]
                }
                frame 14 {
                  w306 = u16 14 items=["氨氮"=3, "水温"=9, "pH"=10, "溶解氧"=11, "电导率"=12, "浊度"=13, "叶绿素a"=14, "藻密度"=15, "蓝绿藻"=16, "氧化还原电位"=17, "溶解氧%"=18, "盐度"=19, "水中油"=20, "高锰酸盐指数"=21, "化学需氧量"=22, "比电导率"=23, "总溶解固体"=24, "pH电极电位"=25] ("下拉列表")
                  n146 = Bundle By Name(cluster=w302, "叶绿素"=1.0 ("DO")) -> (w301:T6)
                  n147 = call "多参数测量数据读取.vi"("探头选择"=w306) -> ("error out"=w295:errorcluster, "测量数据块"=w300:T7)  [unwired: 8 in, 1 out]
                  n148 = case shown="无错误" w295 {
                    tunnel: w300 -> [w307 _]
                    frame No Error {
                      n149 = global write "多参数全局变量.vi" "叶绿素数据区"(w307) -> ()
                    }
                    frame Error {
                    }
                  }
                  n150 = call "多参数据转列表.vi"("参数名"="叶绿素a", "测量数据块"=w300) -> ("添加的数组"=w298:string[][])  [unwired: 9 in]
                  n151 = Index Array(array=w298) -> (element #1=w297:string[], element #2=w296:string[])  [unwired: 4 in]
                  n152 = Insert Into Array(array=w305, new element=w296) -> (w304:string[][])  [unwired: 2 in]
                }
                frame 15 {
                  w319 = u16 15 items=["氨氮"=3, "水温"=9, "pH"=10, "溶解氧"=11, "电导率"=12, "浊度"=13, "叶绿素a"=14, "藻密度"=15, "蓝绿藻"=16, "氧化还原电位"=17, "溶解氧%"=18, "盐度"=19, "水中油"=20, "高锰酸盐指数"=21, "化学需氧量"=22, "比电导率"=23, "总溶解固体"=24, "pH电极电位"=25] ("下拉列表")
                  n153 = call "多参数测量数据读取.vi"("探头选择"=w319) -> ("error out"=w308:errorcluster, "测量数据块"=w311:T7)  [unwired: 8 in, 1 out]
                  n154 = case shown="无错误" w308 {
                    tunnel: w311 -> [w320 _]
                    frame No Error {
                      n155 = global write "多参数全局变量.vi" "藻密度数据区"(w320) -> ()
                    }
                    frame Error {
                    }
                  }
                  n156 = call "多参数据转列表.vi"("参数名"="藻密度", "测量数据块"=w311) -> ("添加的数组"=w313:string[][])  [unwired: 9 in]
                  n157 = Index Array(array=w313) -> (element #1=w312:string[], element #2=w310:string[])  [unwired: 4 in]
                  n158 = Insert Into Array(array=w318, new element=w310) -> (w317:string[][])  [unwired: 2 in]
                  n159 = Bundle By Name(cluster=w315, "藻密度"=1.0 ("DO")) -> (w314:T6)
                }
                frame 16 {
                  w332 = u16 16 items=["氨氮"=3, "水温"=9, "pH"=10, "溶解氧"=11, "电导率"=12, "浊度"=13, "叶绿素a"=14, "藻密度"=15, "蓝绿藻"=16, "氧化还原电位"=17, "溶解氧%"=18, "盐度"=19, "水中油"=20, "高锰酸盐指数"=21, "化学需氧量"=22, "比电导率"=23, "总溶解固体"=24, "pH电极电位"=25] ("下拉列表")
                  n160 = call "多参数测量数据读取.vi"("探头选择"=w332) -> ("error out"=w321:errorcluster, "测量数据块"=w326:T7)  [unwired: 8 in, 1 out]
                  n161 = case shown="无错误" w321 {
                    tunnel: w326 -> [w333 _]
                    frame No Error {
                      n162 = global write "多参数全局变量.vi" "蓝绿藻数据区"(w333) -> ()
                    }
                    frame Error {
                    }
                  }
                  n163 = call "多参数据转列表.vi"("参数名"="蓝绿藻", "测量数据块"=w326) -> ("添加的数组"=w325:string[][])  [unwired: 9 in]
                  n164 = Index Array(array=w325) -> (element #1=w324:string[], element #2=w323:string[])  [unwired: 4 in]
                  n165 = Insert Into Array(array=w331, new element=w323) -> (w330:string[][])  [unwired: 2 in]
                  n166 = Bundle By Name(cluster=w328, "蓝绿藻"=1.0 ("DO")) -> (w327:T6)
                }
                frame 17 {
                  w345 = u16 17 items=["氨氮"=3, "水温"=9, "pH"=10, "溶解氧"=11, "电导率"=12, "浊度"=13, "叶绿素a"=14, "藻密度"=15, "蓝绿藻"=16, "氧化还原电位"=17, "溶解氧%"=18, "盐度"=19, "水中油"=20, "高锰酸盐指数"=21, "化学需氧量"=22, "比电导率"=23, "总溶解固体"=24, "pH电极电位"=25] ("下拉列表")
                  n167 = Bundle By Name(cluster=w341, "ORP"=1.0 ("DO")) -> (w340:T6)
                  n168 = call "多参数测量数据读取.vi"("探头选择"=w345) -> ("error out"=w334:errorcluster, "测量数据块"=w339:T7)  [unwired: 8 in, 1 out]
                  n169 = case shown="无错误" w334 {
                    tunnel: w339 -> [w346 _]
                    frame No Error {
                      n170 = global write "多参数全局变量.vi" "ORP数据区"(w346) -> ()
                    }
                    frame Error {
                    }
                  }
                  n171 = call "多参数据转列表.vi"("参数名"="ORP", "测量数据块"=w339) -> ("添加的数组"=w338:string[][])  [unwired: 9 in]
                  n172 = Index Array(array=w338) -> (element #1=w337:string[], element #2=w335:string[])  [unwired: 4 in]
                  n173 = Insert Into Array(array=w344, new element=w335) -> (w343:string[][])  [unwired: 2 in]
                }
                frame 20 {
                  w355 = u16 20 items=["氨氮"=3, "水温"=9, "pH"=10, "溶解氧"=11, "电导率"=12, "浊度"=13, "叶绿素a"=14, "藻密度"=15, "蓝绿藻"=16, "氧化还原电位"=17, "溶解氧%"=18, "盐度"=19, "水中油"=20, "高锰酸盐指数"=21, "化学需氧量"=22, "比电导率"=23, "总溶解固体"=24, "pH电极电位"=25] ("下拉列表")
                  n174 = call "多参数测量数据读取.vi"("探头选择"=w355) -> ("测量数据块"=w351:T7)  [unwired: 8 in, 2 out]
                  n175 = call "多参数据转列表.vi"("参数名"="水中油", "测量数据块"=w351) -> ("添加的数组"=w349:string[][])  [unwired: 9 in]
                  n176 = Index Array(array=w349) -> (element #1=w348:string[], element #2=w347:string[])  [unwired: 4 in]
                  n177 = Insert Into Array(array=w354, new element=w347) -> (w353:string[][])  [unwired: 2 in]
                }
                frame 21 {
                  w364 = u16 21 items=["氨氮"=3, "水温"=9, "pH"=10, "溶解氧"=11, "电导率"=12, "浊度"=13, "叶绿素a"=14, "藻密度"=15, "蓝绿藻"=16, "氧化还原电位"=17, "溶解氧%"=18, "盐度"=19, "水中油"=20, "高锰酸盐指数"=21, "化学需氧量"=22, "比电导率"=23, "总溶解固体"=24, "pH电极电位"=25] ("下拉列表")
                  n178 = call "多参数测量数据读取.vi"("探头选择"=w364) -> ("测量数据块"=w360:T7)  [unwired: 8 in, 2 out]
                  n179 = call "多参数据转列表.vi"("参数名"="高锰酸盐指数", "测量数据块"=w360) -> ("添加的数组"=w359:string[][])  [unwired: 9 in]
                  n180 = Index Array(array=w359) -> (element #1=w357:string[], element #2=w356:string[])  [unwired: 4 in]
                  n181 = Insert Into Array(array=w363, new element=w356) -> (w362:string[][])  [unwired: 2 in]
                }
                frame 22 {
                  w373 = u16 22 items=["氨氮"=3, "水温"=9, "pH"=10, "溶解氧"=11, "电导率"=12, "浊度"=13, "叶绿素a"=14, "藻密度"=15, "蓝绿藻"=16, "氧化还原电位"=17, "溶解氧%"=18, "盐度"=19, "水中油"=20, "高锰酸盐指数"=21, "化学需氧量"=22, "比电导率"=23, "总溶解固体"=24, "pH电极电位"=25] ("下拉列表")
                  n182 = call "多参数测量数据读取.vi"("探头选择"=w373) -> ("测量数据块"=w369:T7)  [unwired: 8 in, 2 out]
                  n183 = call "多参数据转列表.vi"("参数名"="化学需氧量", "测量数据块"=w369) -> ("添加的数组"=w368:string[][])  [unwired: 9 in]
                  n184 = Index Array(array=w368) -> (element #1=w366:string[], element #2=w365:string[])  [unwired: 4 in]
                  n185 = Insert Into Array(array=w372, new element=w365) -> (w371:string[][])  [unwired: 2 in]
                }
              }
            }
            n186 = global write "多参数全局变量.vi" "传感器通道号"(w147) -> ()
            n187 = property on="数据区" class="MCListbox (严格)"("ColHdrString"=w153, "ItemNames"=w152) -> ()  [unwired: 2 in, 2 out]
          }
          frame Error {
          }
        }
      }
    }
    n188 = Wait (ms)(milliseconds to wait=u32 1000 ("等待时间（毫秒）")) -> ()  [unwired: 1 out]
  }
  n189 = property on="窗格" class="Pane"("Origin"=T3 {"Horizontal"=0, "Vertical"=0} ("原点")) -> ()  [unwired: 2 in, 2 out]
  n190 = property class="VI"(reference=w8) -> ("Library.Version"=w7:T8)  [unwired: 1 in, 2 out]
  n191 = call <vilib>:"Application Directory.vi"() -> ("Application Directory"=w14:path)
  n192 = Build Path(base path=w14, name or relative path="data\\sys.ini" ("名称或相对路径")) -> (appended path=w16:path)
  n193 = Unbundle By Name(w7) -> ("Major"=w5:u16, "Minor"=w4:u16, "Fix"=w3:u16, "Build"=w2:u16)
  n194 = call <vilib>:"Open Config Data.vi"("configuration file path"=w16) -> ("error out"=w20:errorcluster, "refnum"=w17:T9)  [unwired: 8 in, 1 out]
  n195 = vi-ref "多参数断电保存全局变量.vi"() -> (w18:refnum<vi>)
  n196 = call <userlib>:"Read Panel from INI__ogtk.vi"("error in (no error)"=w20, "VI ref"=w18, "refnum"=w17) -> ("error out"=w21:errorcluster, "refnum out"=w19:T9)  [unwired: 7 in]
  n197 = Obtain Queue(name (unnamed)="Mp Task" ("名称（未命名）"), element data type=T2 {"测量模式"="", "数据类型"="N"} ("启动参数")) -> (queue out=w9:refnum<queue>)  [unwired: 3 in, 2 out]
  n198 = property on="打开串口" class="Bool (严格)"("Val(Sgnl)"=TRUE ("值(信号)")) -> (error out=w22:errorcluster)  [unwired: 2 in, 1 out]
  n199 = call <vilib>:"Close Config Data.vi"("error in (no error)"=w21, "refnum"=w19) -> ("error out"=w13:errorcluster)  [unwired: 8 in, 1 out]
  n200 = Format Into String(format string="模块版本号：%d.%d.%d.%d" ("格式字符串"), w5, w4, w3, w2) -> (resulting string=→"模块版本号":string)  [unwired: 2 in, 1 out]
  n201 = Obtain Notifier(name (unnamed)="MPFlow" ("名称（未命名）"), notification data type=FALSE) -> (notifier out=w25:refnum<notifier>)  [unwired: 2 in, 2 out]
  n202 = while {
    tunnel: w9 -> [w375]
    stop <- FALSE stop-if-true
    n203 = flat-sequence {
      tunnel: w375 -> [w379]
      tunnel: [w377] -> w374
      frame #0 {
        n204 = Dequeue Element(queue=w379) -> (queue out=w377:refnum<queue>, element=w378:T2)  [unwired: 2 in, 2 out]
        n205 = call "五参数水样测试.vi"("启动参数"=w378) -> ()  [unwired: 11 in]
      }
    }
    n206 = Flush Queue(queue=w374) -> ()  [unwired: 1 in, 3 out]
  }
  n207 = vi-ref "五参数标样核查.vi"() -> (w12:refnum<vi>)
  n208 = control-ref of="控制命令区探头选择"() -> (w24:refnum<vi>)
  n209 = while {
    tunnel: w25 -> [w383]
    tunnel: w24 -> [w382]
    tunnel: w22 -> [_]
    tunnel: w13 -> [_]
    tunnel: w12 -> [w381]
    tunnel: w9 -> [w380]
    stop <- FALSE stop-if-true
    n210 = event shown="[13] \"标样核查\": 值改变" {
      selector: _ -> [_ _ _ _ _ _ _ _ _ _ _ _ _ _ _ _ _ _ _ _ _ _ _ _ _]
      dyn-events: _ -> [_ _ _ _ _ _ _ _ _ _ _ _ _ _ _ _ _ _ _ _ _ _ _ _ _]
      timeout: _ -> [_ _ _ _ _ _ _ _ _ _ _ _ _ _ _ _ _ _ _ _ _ _ _ _ _]
      tunnel: w383 -> [_ _ _ _ _ _ _ _ _ _ _ _ _ _ w535 _ _ _ _ _ _ _ _ _ _]
      tunnel: w382 -> [_ _ w392 w396 _ _ _ _ _ _ _ _ _ _ _ _ _ _ _ _ _ _ _ w592 w599]
      tunnel: w381 -> [_ _ _ _ _ _ _ _ _ _ _ _ _ w511 _ _ _ _ _ _ _ _ _ _ _]
      tunnel: w380 -> [_ _ _ _ _ _ _ _ _ _ _ _ w507 _ _ _ _ _ _ _ _ _ _ _ _]
      event Timeout {
        n211 = event-data() -> ()  [unwired: 1 in, 3 out]
      }
      event "K", "B", "水深校准", "水样稳定时间", "上电初始化时间", "转刷清洗时间", "水样测试组数", "标样测试组数": Mouse Down {
        n212 = event-data() -> ("CtlRef"=w388:refnum<vi>)  [unwired: 1 in, 7 out]
        n213 = property class="DigNum (严格)"(reference=w388) -> (reference out=w386:refnum<vi>, "Value"=w387:dbl)  [unwired: 1 in, 1 out]
        n214 = call "数字键盘.vi"("OldNumber"=w387) -> ("NewNumber"=w385:dbl)
        n215 = property class="DigNum (严格)"(reference=w386, "Value"=w385) -> ()  [unwired: 1 in, 2 out]
      }
      event "读取": Value Change {
        n216 = event-data() -> ()  [unwired: 1 in, 6 out]
        n217 = property class="Ring (严格)"(reference=w392) -> ("Value"=w391:u16)  [unwired: 1 in, 2 out]
        n218 = call "多参校准读取.vi"("站号"=w391) -> ("B"=w389:dbl, "K"=w390:dbl)  [unwired: 8 in, 1 out]
        n219 = local write "K"(w390) -> ()
        n220 = local write "B"(w389) -> ()
      }
      event "写入": Value Change {
        n221 = event-data() -> ()  [unwired: 1 in, 6 out]
        n222 = property class="Ring (严格)"(reference=w396) -> ("Value"=w395:u16)  [unwired: 1 in, 2 out]
        n223 = call "多参数校准写入.vi"("B"="B", "K"="K", "站号"=w395) -> ()  [unwired: 8 in, 1 out]
      }
      event "水深读取": Value Change {
        w398 = u16 9 items=["氨氮"=3, "水温"=9, "pH值"=10, "溶解氧"=11, "电导率"=12, "浊度"=13, "叶绿素a"=14, "藻密度"=15, "蓝绿藻"=16, "氧化还原电位"=17, "溶解氧%"=18, "盐度"=19] ("站号")
        n224 = event-data() -> ()  [unwired: 1 in, 6 out]
        n225 = call "多参水深校准读取.vi"("站号"=w398) -> ("B"=w397:dbl)  [unwired: 8 in, 2 out]
        n226 = local write "水深校准"(w397) -> ()
      }
      event "水深写入": Value Change {
        w400 = u16 9 items=["氨氮"=3, "水温"=9, "pH值"=10, "溶解氧"=11, "电导率"=12, "浊度"=13, "叶绿素a"=14, "藻密度"=15, "蓝绿藻"=16, "氧化还原电位"=17, "溶解氧%"=18, "盐度"=19] ("站号")
        n227 = event-data() -> ()  [unwired: 1 in, 6 out]
        n228 = call "多参数水深校准写入.vi"("K"="水深校准", "站号"=w400) -> ()  [unwired: 9 in, 1 out]
      }
      event "串口设置": Value Change {
        n229 = event-data() -> ()  [unwired: 1 in, 6 out]
        n230 = global read "多参数断电保存全局变量.vi" "VISA Resource"() -> (w405:refnum<visa-resource-name>)
        n231 = global read "多参数断电保存全局变量.vi" "波特率"() -> (w403:u32)
        n232 = call "串口配置.vi"("波特率"=w403, "VISA资源名称"=w405) -> ("确认 2"=w401:bool, "波特率 2"=w402:u32, "VISA资源名称 2"=w404:refnum<visa-resource-name>)  [unwired: 7 in]
        n233 = case shown="真" w401 {
          tunnel: w404 -> [_ w407]
          tunnel: w402 -> [_ w406]
          frame False {
          }
          frame True {
            n234 = flat-sequence {
              tunnel: w407 -> [w409]
              tunnel: w406 -> [w408]
              frame #0 {
                n235 = global write "多参数断电保存全局变量.vi" "VISA Resource"(w409) -> ()
                n236 = global write "多参数断电保存全局变量.vi" "波特率"(w408) -> ()
              }
              frame #1 {
                n237 = call "多参数通讯.vi"("STEP"=enum16{"open", "read", "write", "close"}."open") -> ("error out"=w411:errorcluster)  [unwired: 8 in, 2 out]
                n238 = case shown="错误" w411 {
                  frame No Error {
                  }
                  frame Error {
                    n239 = One Button Dialog(message="多参数串口打开失败" ("消息")) -> ()  [unwired: 1 in, 1 out]
                  }
                }
              }
              frame #2 {
                n240 = call <vilib>:"Application Directory.vi"() -> ("Application Directory"=w426:path)
                n241 = Build Path(base path=w426, name or relative path="data\\sys.ini" ("名称或相对路径")) -> (appended path=w424:path)
                n242 = call <vilib>:"Open Config Data.vi"("configuration file path"=w424) -> ("error out"=w420:errorcluster, "refnum"=w423:T9)  [unwired: 8 in, 1 out]
                n243 = vi-ref "多参数断电保存全局变量.vi"() -> (w422:refnum<vi>)
                n244 = call <userlib>:"Write Panel to INI__ogtk.vi"("error in (no error)"=w420, "VI ref"=w422, "refnum"=w423) -> ("error out"=w419:errorcluster, "refnum out"=w421:T9)  [unwired: 7 in]
                n245 = call <vilib>:"Close Config Data.vi"("error in (no error)"=w419, "refnum"=w421) -> ("error out"=w414:errorcluster, "file path"=w413:path)  [unwired: 8 in]
                n246 = Open/Create/Replace File(file path (use dialog)=w413, error in=w414) -> (refnum out=w417:refnum<file>, error out=w418:errorcluster)  [unwired: 4 in, 1 out]
                n247 = Flush File(refnum=w417, error in=w418) -> (refnum out=w416:refnum<file>, error out=w415:errorcluster)
                n248 = Close File(refnum=w416, error in=w415) -> ()  [unwired: 2 out]
              }
            }
          }
        }
      }
      event "水样稳定时间", "上电初始化时间", "转刷清洗时间", "水样测试组数", "标样测试组数": Value Change {
        n249 = event-data() -> ()  [unwired: 1 in, 6 out]
        n250 = flat-sequence {
          frame #0 {
            n251 = global write "多参数断电保存全局变量.vi" "水样稳定时间"("水样稳定时间") -> ()
            n252 = global write "多参数断电保存全局变量.vi" "水样测试组数"("水样测试组数") -> ()
            n253 = global write "多参数断电保存全局变量.vi" "上电初始化时间"("上电初始化时间") -> ()
            n254 = global write "多参数断电保存全局变量.vi" "转刷清洗时间"("转刷清洗时间") -> ()
            n255 = global write "多参数断电保存全局变量.vi" "标样测试组数"("标样测试组数") -> ()
          }
          frame #1 {
            n256 = call <vilib>:"Application Directory.vi"() -> ("Application Directory"=w445:path)
            n257 = Build Path(base path=w445, name or relative path="data\\sys.ini" ("名称或相对路径")) -> (appended path=w443:path)
            n258 = call <vilib>:"Open Config Data.vi"("configuration file path"=w443) -> ("error out"=w439:errorcluster, "refnum"=w442:T9)  [unwired: 8 in, 1 out]
            n259 = vi-ref "多参数断电保存全局变量.vi"() -> (w441:refnum<vi>)
            n260 = call <userlib>:"Write Panel to INI__ogtk.vi"("error in (no error)"=w439, "VI ref"=w441, "refnum"=w442) -> ("error out"=w438:errorcluster, "refnum out"=w440:T9)  [unwired: 7 in]
            n261 = call <vilib>:"Close Config Data.vi"("error in (no error)"=w438, "refnum"=w440) -> ("error out"=w433:errorcluster, "file path"=w432:path)  [unwired: 8 in]
            n262 = Open/Create/Replace File(file path (use dialog)=w432, error in=w433) -> (refnum out=w436:refnum<file>, error out=w437:errorcluster)  [unwired: 4 in, 1 out]
            n263 = Flush File(refnum=w436, error in=w437) -> (refnum out=w435:refnum<file>, error out=w434:errorcluster)
            n264 = Close File(refnum=w435, error in=w434) -> ()  [unwired: 2 out]
          }
        }
      }
      event "传感器参数自动获取": Value Change {
        n265 = event-data() -> ("NewVal"=w446:bool)  [unwired: 1 in, 5 out]
        n266 = case shown="假" w446 {
          frame False {
            n267 = property on="获取传感器参数并保存触发" class="Bool (严格)"("Val(Sgnl)"=FALSE ("获取传感器参数并保存触发")) -> ()  [unwired: 2 in, 2 out]
          }
          frame True {
          }
        }
        n268 = flat-sequence {
          tunnel: w446 -> [w448]
          frame #0 {
            n269 = global write "多参数断电保存全局变量.vi" "传感器参数自动获取"(w448) -> ()
          }
          frame #1 {
            n270 = call <vilib>:"Application Directory.vi"() -> ("Application Directory"=w462:path)
            n271 = Build Path(base path=w462, name or relative path="data\\sys.ini" ("名称或相对路径")) -> (appended path=w460:path)
            n272 = call <vilib>:"Open Config Data.vi"("configuration file path"=w460) -> ("error out"=w456:errorcluster, "refnum"=w459:T9)  [unwired: 8 in, 1 out]
            n273 = vi-ref "多参数断电保存全局变量.vi"() -> (w458:refnum<vi>)
            n274 = call <userlib>:"Write Panel to INI__ogtk.vi"("error in (no error)"=w456, "VI ref"=w458, "refnum"=w459) -> ("error out"=w455:errorcluster, "refnum out"=w457:T9)  [unwired: 7 in]
            n275 = call <vilib>:"Close Config Data.vi"("error in (no error)"=w455, "refnum"=w457) -> ("error out"=w450:errorcluster, "file path"=w449:path)  [unwired: 8 in]
            n276 = Open/Create/Replace File(file path (use dialog)=w449, error in=w450) -> (refnum out=w453:refnum<file>, error out=w454:errorcluster)  [unwired: 4 in, 1 out]
            n277 = Flush File(refnum=w453, error in=w454) -> (refnum out=w452:refnum<file>, error out=w451:errorcluster)
            n278 = Close File(refnum=w452, error in=w451) -> ()  [unwired: 2 out]
          }
        }
      }
      event "质控参数设置": Value Change {
        n279 = event-data() -> ()  [unwired: 1 in, 6 out]
        n280 = global read "多参数断电保存全局变量.vi" "质控参数设置"() -> (w463:T12)
        n281 = call "多参数质控参数设置.vi"("质控参数设置"=w463) -> ("输出簇"=w464:T13)  [unwired: 10 in]
        n282 = Unbundle By Name(w464) -> ("确定"=w465:bool)
        n283 = case shown="真" w465 {
          tunnel: w464 -> [_ w467]
          tunnel: w463 -> [_ w466]
          frame False {
          }
          frame True {
            n284 = flat-sequence {
              tunnel: w467 -> [w475]
              tunnel: w466 -> [w474]
              frame #0 {
                n285 = Unbundle By Name(w475) -> ("水温标准液标准浓度"=w473:dbl, "酸碱度标准液标准浓度"=w472:dbl, "溶解氧标准液标准浓度"=w471:dbl, "电导率标准液标准浓度"=w470:dbl, "浊度标准液标准浓度"=w469:dbl)
                n286 = Bundle By Name(cluster=w474, "水温标准液标准浓度"=w473, "酸碱度标准液标准浓度"=w472, "溶解氧标准液标准浓度"=w471, "电导率标准液标准浓度"=w470, "浊度标准液标准浓度"=w469) -> (w468:T12)
                n287 = global write "多参数断电保存全局变量.vi" "质控参数设置"(w468) -> ()
              }
              frame #1 {
                n288 = call <vilib>:"Application Directory.vi"() -> ("Application Directory"=w489:path)
                n289 = Build Path(base path=w489, name or relative path="data\\sys.ini" ("名称或相对路径")) -> (appended path=w487:path)
                n290 = call <vilib>:"Open Config Data.vi"("configuration file path"=w487) -> ("error out"=w483:errorcluster, "refnum"=w486:T9)  [unwired: 8 in, 1 out]
                n291 = vi-ref "多参数断电保存全局变量.vi"() -> (w485:refnum<vi>)
                n292 = call <userlib>:"Write Panel to INI__ogtk.vi"("error in (no error)"=w483, "VI ref"=w485, "refnum"=w486) -> ("error out"=w482:errorcluster, "refnum out"=w484:T9)  [unwired: 7 in]
                n293 = call <vilib>:"Close Config Data.vi"("error in (no error)"=w482, "refnum"=w484) -> ("error out"=w477:errorcluster, "file path"=w476:path)  [unwired: 8 in]
                n294 = Open/Create/Replace File(file path (use dialog)=w476, error in=w477) -> (refnum out=w480:refnum<file>, error out=w481:errorcluster)  [unwired: 4 in, 1 out]
                n295 = Flush File(refnum=w480, error in=w481) -> (refnum out=w479:refnum<file>, error out=w478:errorcluster)
                n296 = Close File(refnum=w479, error in=w478) -> ()  [unwired: 2 out]
              }
            }
          }
        }
      }
      event "释放串口": Value Change {
        n297 = event-data() -> ("NewVal"=w490:bool)  [unwired: 1 in, 5 out]
        n298 = case shown="真" w490 {
          frame False {
          }
          frame True {
            n299 = call "多参数通讯.vi"("STEP"=enum16{"open", "read", "write", "close"}."close") -> ("error out"=w491:errorcluster)  [unwired: 8 in, 2 out]
            n300 = case shown="无错误" w491 {
              frame No Error {
                n301 = property on="打开串口" class="Bool (严格)"("DisabledEnum"=T10."Enabled" ("禁用")) -> ()  [unwired: 2 in, 2 out]
              }
              frame Error {
              }
            }
          }
        }
      }
      event "打开串口": Value Change {
        n302 = event-data() -> ("NewVal"=w494:bool)  [unwired: 1 in, 5 out]
        n303 = case shown="真" w494 {
          frame False {
          }
          frame True {
            n304 = call "多参数通讯.vi"("STEP"=enum16{"open", "read", "write", "close"}."open") -> ("error out"=w495:errorcluster)  [unwired: 8 in, 2 out]
            n305 = case shown="错误" w495 {
              tunnel: [T10."Disabled and Grayed Out" ("禁用") T10."Enabled" ("禁用")] -> w497
              frame No Error {
              }
              frame Error {
                n306 = One Button Dialog(message="多参数串口打开失败" ("消息")) -> ()  [unwired: 1 in, 1 out]
              }
            }
            n307 = property on="打开串口" class="Bool (严格)"("DisabledEnum"=w497, "Value"=FALSE ("打开串口")) -> ()  [unwired: 2 in, 2 out]
          }
        }
      }
      event "水样测试": Value Change {
        n308 = event-data() -> ()  [unwired: 1 in, 6 out]
        n309 = global read "多参数断电保存全局变量.vi" "运行周期"() -> (w505:T14)
        n310 = Unbundle By Name(w505) -> ("运行模式"=w504:enum16{"维护模式", "常规模式", "应急模式", "质控模式"})
        n311 = case shown="\"维护模式\"" w504 {
          tunnel: ["M" ("数据类型") "hd" ("数据类型")] -> w502
          frame "维护模式" {
          }
          frame "常规模式", Default {
          }
        }
        n312 = Bundle By Name(cluster=T2 {"测量模式"="水样测试", "数据类型"="N"} ("启动参数"), "数据类型"=w502) -> (w503:T2)
        n313 = Enqueue Element(queue=w507, element=w503) -> ()  [unwired: 2 in, 3 out]
      }
      event "标样核查": Value Change {
        n314 = event-data() -> ()  [unwired: 1 in, 6 out]
        n315 = call "多参数标样核查对话框.vi"() -> ("确认"=w512:bool, "输出参数"=w510:T15)  [unwired: 10 in]
        n316 = case shown="真" w512 {
          tunnel: w511 -> [_ w515]
          tunnel: w510 -> [_ w514]
          frame False {
          }
          frame True {
            n317 = property class="VI"(reference=w515) -> ("Name"=w519:string, "Exec.State"=w517:T16)  [unwired: 1 in, 2 out]
            n318 = Open VI Reference(type specifier VI Refnum (for type only)=refnum<vi> refnum, vi path=w519, options=128 ("选项")) -> (vi reference=w518:refnum<vi>)  [unwired: 3 in, 1 out]
            n319 = case shown="\"Idle\"" w517 {
              tunnel: w518 -> [w522 w530]
              tunnel: [w522 w529] -> w516
              tunnel: w514 -> [_ w527]
              frame "Bad", Default {
                n320 = One Button Dialog(message="仪器已经启动，无需重复启动" ("消息")) -> ()  [unwired: 1 in, 1 out]
              }
              frame "Idle" {
                n321 = global read "多参数断电保存全局变量.vi" "运行周期"() -> (w526:T14)
                n322 = Unbundle By Name(w526) -> ("运行模式"=w525:enum16{"维护模式", "常规模式", "应急模式", "质控模式"})
                n323 = case shown="\"维护模式\"" w525 {
                  tunnel: ["M" ("数据标记表") "N" ("数据标记表")] -> w528
                  frame "维护模式" {
                  }
                  frame "常规模式", Default {
                  }
                }
                n324 = Bundle By Name(cluster=T11 {"测量模式"="标样核查", "数据类型"="N", "输出参数"={"水温"=FALSE, "pH"=FALSE, "DO"=FALSE, "浊度"=FALSE, "电导率"=FALSE}} ("启动参数"), "数据类型"=w528, "输出参数"=w527) -> (w523:T11)
                n325 = call-by-ref "开始异步调用"(reference=w530, "启动参数"=w523) -> (reference out=w529:refnum<vi>)  [unwired: 12 in, 1 out]
              }
            }
            n326 = Close Reference(reference=w516) -> ()  [unwired: 1 in, 1 out]
          }
        }
      }
      event "停止": Value Change {
        n327 = event-data() -> ()  [unwired: 1 in, 6 out]
        n328 = Two Button Dialog(message="请再一次确认是否停止测量" ("消息")) -> (T button?=w533:bool)  [unwired: 2 in]
        n329 = case shown="真" w533 {
          tunnel: w535 -> [_ w538]
          frame False {
          }
          frame True {
            w536 = u16 11 items=["启动测量（全部）"=1, "初始化（清洗）"=10, "停止测量（全部）"=11, "校时"=13, "启动测量（单个传感器）"=19, "停止测量（单个传感器）"=20] ("控制命令")
            w537 = u16 10 items=["氨氮"=3, "水温"=9, "pH值"=10, "溶解氧"=11, "电导率"=12, "浊度"=13, "叶绿素a"=14, "藻密度"=15, "蓝绿藻"=16, "氧化还原电位"=17, "溶解氧%"=18, "盐度"=19] ("站号")
            n330 = Send Notification(notification=TRUE ("通知"), notifier=w538) -> ()  [unwired: 1 in, 2 out]
            n331 = call "多参数控制命令.vi"("控制命令"=w536, "站号"=w537) -> ()  [unwired: 9 in, 1 out]
          }
        }
      }
      event "设置": Value Change {
        n332 = event-data() -> ()  [unwired: 1 in, 6 out]
        n333 = property on="窗格" class="Pane"("Origin"=T3 {"Horizontal"=0, "Vertical"=628} ("原点")) -> ()  [unwired: 2 in, 2 out]
      }
      event "返回": Value Change {
        n334 = event-data() -> ()  [unwired: 1 in, 6 out]
        n335 = property on="窗格" class="Pane"("Origin"=T3 {"Horizontal"=0, "Vertical"=0} ("原点")) -> ()  [unwired: 2 in, 2 out]
      }
      event "传感器参数读取", "获取传感器参数并保存触发": Value Change {
        n336 = event-data() -> ()  [unwired: 1 in, 6 out]
        n337 = call "多参数传感器参数读取.vi"() -> ("error out"=w545:errorcluster, "modbus"=w543:u16[], "添加的数组"=w544:string[][])  [unwired: 9 in]
        n338 = property on="传感器区" class="MCListbox (严格)"("ItemNames"=w544) -> ()  [unwired: 2 in, 2 out]
        n339 = call <vilib>:"General Error Handler.vi"("error in (no error)"=w545) -> ("error out"=w542:errorcluster)  [unwired: 10 in, 4 out]
        n340 = case shown="无错误" w542 {
          tunnel: w543 -> [w546 _]
          frame No Error {
            n341 = flat-sequence {
              tunnel: w546 -> [w547]
              frame #0 {
                n342 = global write "多参数断电保存全局变量.vi" "传感器参数modbus"(w547) -> ()
              }
              frame #1 {
                n343 = call <vilib>:"Application Directory.vi"() -> ("Application Directory"=w561:path)
                n344 = Build Path(base path=w561, name or relative path="data\\sys.ini" ("名称或相对路径")) -> (appended path=w559:path)
                n345 = call <vilib>:"Open Config Data.vi"("configuration file path"=w559) -> ("error out"=w555:errorcluster, "refnum"=w558:T9)  [unwired: 8 in, 1 out]
                n346 = vi-ref "多参数断电保存全局变量.vi"() -> (w557:refnum<vi>)
                n347 = call <userlib>:"Write Panel to INI__ogtk.vi"("error in (no error)"=w555, "VI ref"=w557, "refnum"=w558) -> ("error out"=w554:errorcluster, "refnum out"=w556:T9)  [unwired: 7 in]
                n348 = call <vilib>:"Close Config Data.vi"("error in (no error)"=w554, "refnum"=w556) -> ("error out"=w549:errorcluster, "file path"=w548:path)  [unwired: 8 in]
                n349 = Open/Create/Replace File(file path (use dialog)=w548, error in=w549) -> (refnum out=w552:refnum<file>, error out=w553:errorcluster)  [unwired: 4 in, 1 out]
                n350 = Flush File(refnum=w552, error in=w553) -> (refnum out=w551:refnum<file>, error out=w550:errorcluster)
                n351 = Close File(refnum=w551, error in=w550) -> ()  [unwired: 2 out]
              }
            }
          }
          frame Error {
          }
        }
      }
      event "关键参数区读取": Value Change {
        n352 = event-data() -> ()  [unwired: 1 in, 6 out]
        n353 = call "多参数关键参数读取.vi"() -> ("error out"=w562:errorcluster, "添加的数组"=w563:string[][])  [unwired: 10 in]
        n354 = property on="关键参数区" class="MCListbox (严格)"("ItemNames"=w563) -> ()  [unwired: 2 in, 2 out]
        n355 = call <vilib>:"General Error Handler.vi"("error in (no error)"=w562) -> ()  [unwired: 10 in, 5 out]
      }
      event "同步时间": Value Change {
        w564 = u16 13 items=["启动测量（全部）"=1, "初始化（清洗）"=10, "停止测量（全部）"=11, "校时"=13, "启动测量（单个传感器）"=19, "停止测量（单个传感器）"=20] ("控制命令")
        w565 = u16 9 items=["氨氮"=3, "水温"=9, "pH值"=10, "溶解氧"=11, "电导率"=12, "浊度"=13, "叶绿素a"=14, "藻密度"=15, "蓝绿藻"=16, "氧化还原电位"=17, "溶解氧%"=18, "盐度"=19] ("站号")
        n356 = event-data() -> ()  [unwired: 1 in, 6 out]
        n357 = call "多参数控制命令.vi"("控制命令"=w564, "站号"=w565) -> ("error out"=w567:errorcluster)  [unwired: 9 in]
        n358 = case shown="错误" w567 {
          tunnel: ["时间同步成功" ("消息") "时间同步失败" ("消息")] -> w566
          frame No Error {
          }
          frame Error {
          }
        }
        n359 = One Button Dialog(message=w566) -> ()  [unwired: 1 in, 1 out]
      }
      event "启动测量(全部)": Value Change {
        w570 = u16 1 items=["启动测量（全部）"=1, "初始化（清洗）"=10, "停止测量（全部）"=11, "校时"=13, "启动测量（单个传感器）"=19, "停止测量（单个传感器）"=20] ("控制命令")
        w571 = u16 9 items=["氨氮"=3, "水温"=9, "pH值"=10, "溶解氧"=11, "电导率"=12, "浊度"=13, "叶绿素a"=14, "藻密度"=15, "蓝绿藻"=16, "氧化还原电位"=17, "溶解氧%"=18, "盐度"=19] ("站号")
        n360 = event-data() -> ()  [unwired: 1 in, 6 out]
        n361 = call "多参数控制命令.vi"("控制命令"=w570, "站号"=w571) -> ("error out"=w573:errorcluster)  [unwired: 9 in]
        n362 = case shown="无错误" w573 {
          tunnel: ["启动成功" ("消息") "启动失败" ("消息")] -> w572
          frame No Error {
          }
          frame Error {
          }
        }
        n363 = One Button Dialog(message=w572) -> ()  [unwired: 1 in, 1 out]
      }
      event "停止测量(全部)": Value Change {
        w578 = u16 11 items=["启动测量（全部）"=1, "初始化（清洗）"=10, "停止测量（全部）"=11, "校时"=13, "启动测量（单个传感器）"=19, "停止测量（单个传感器）"=20] ("控制命令")
        w579 = u16 9 items=["氨氮"=3, "水温"=9, "pH值"=10, "溶解氧"=11, "电导率"=12, "浊度"=13, "叶绿素a"=14, "藻密度"=15, "蓝绿藻"=16, "氧化还原电位"=17, "溶解氧%"=18, "盐度"=19] ("站号")
        n364 = event-data() -> ()  [unwired: 1 in, 6 out]
        n365 = call "多参数控制命令.vi"("控制命令"=w578, "站号"=w579) -> ("error out"=w577:errorcluster)  [unwired: 9 in]
        n366 = case shown="错误" w577 {
          tunnel: ["停止成功" ("消息") "停止失败" ("消息")] -> w576
          frame No Error {
          }
          frame Error {
          }
        }
        n367 = One Button Dialog(message=w576) -> ()  [unwired: 1 in, 1 out]
      }
      event "初始化(清洗)": Value Change {
        w584 = u16 10 items=["启动测量（全部）"=1, "初始化（清洗）"=10, "停止测量（全部）"=11, "校时"=13, "启动测量（单个传感器）"=19, "停止测量（单个传感器）"=20] ("控制命令")
        w585 = u16 9 items=["氨氮"=3, "水温"=9, "pH值"=10, "溶解氧"=11, "电导率"=12, "浊度"=13, "叶绿素a"=14, "藻密度"=15, "蓝绿藻"=16, "氧化还原电位"=17, "溶解氧%"=18, "盐度"=19] ("站号")
        n368 = event-data() -> ()  [unwired: 1 in, 6 out]
        n369 = call "多参数控制命令.vi"("控制命令"=w584, "站号"=w585) -> ("error out"=w582:errorcluster)  [unwired: 9 in]
        n370 = case shown="错误" w582 {
          tunnel: ["初始化成功" ("消息") "初始化失败" ("消息")] -> w583
          frame No Error {
          }
          frame Error {
          }
        }
        n371 = One Button Dialog(message=w583) -> ()  [unwired: 1 in, 1 out]
      }
      event "启动测量(单探)": Value Change {
        w588 = u16 19 items=["启动测量（全部）"=1, "初始化（清洗）"=10, "停止测量（全部）"=11, "校时"=13, "启动测量（单个传感器）"=19, "停止测量（单个传感器）"=20] ("控制命令")
        n372 = event-data() -> ()  [unwired: 1 in, 6 out]
        n373 = property class="Ring (严格)"(reference=w592) -> ("Value"=w591:u16)  [unwired: 1 in, 2 out]
        n374 = call "多参数控制命令.vi"("控制命令"=w588, "站号"=w591) -> ("error out"=w590:errorcluster)  [unwired: 9 in]
        n375 = case shown="无错误" w590 {
          tunnel: ["启动成功" ("消息") "启动失败" ("消息")] -> w589
          frame No Error {
          }
          frame Error {
          }
        }
        n376 = One Button Dialog(message=w589) -> ()  [unwired: 1 in, 1 out]
      }
      event "停止测量(单探)": Value Change {
        w595 = u16 20 items=["启动测量（全部）"=1, "初始化（清洗）"=10, "停止测量（全部）"=11, "校时"=13, "启动测量（单个传感器）"=19, "停止测量（单个传感器）"=20] ("控制命令")
        n377 = event-data() -> ()  [unwired: 1 in, 6 out]
        n378 = property class="Ring (严格)"(reference=w599) -> ("Value"=w598:u16)  [unwired: 1 in, 2 out]
        n379 = call "多参数控制命令.vi"("控制命令"=w595, "站号"=w598) -> ("error out"=w597:errorcluster)  [unwired: 9 in]
        n380 = case shown="错误" w597 {
          tunnel: ["停止成功" ("消息") "停止失败" ("消息")] -> w596
          frame No Error {
          }
          frame Error {
          }
        }
        n381 = One Button Dialog(message=w596) -> ()  [unwired: 1 in, 1 out]
      }
    }
  }
